vi "dlcTAF.vi"() -> ()   [LabVIEW 2019]
uses:
  <vilib>/DAQmx/write.llb/DAQmx Write (Digital 1D Bool NChan 1Samp 1Line).vi
  <vilib>/DAQmx/write.llb/DAQmx Write (Analog 1D DBL 1Chan NSamp).vi
  <vilib>/DAQmx/read.llb/DAQmx Read (Analog 2D I16 NChan NSamp).vi
  <vilib>/Analysis/baseanly.llb/Mean (DBL).vi
  Instance           1 17Saved   evtaf_amp .vi
  <vilib>/Utility/config.llb/Read Key (Path).vi
  <vilib>/Utility/config.llb/Read Key (String).vi
  <vilib>/Utility/config.llb/Read Key (I32).vi
  <vilib>/Utility/config.llb/Read Key (Double).vi
  <vilib>/Utility/config.llb/Read Key (U32).vi
  Instance           2 17Saved   evtaf_amp .vi
  Instance           3 17Saved   evtaf_amp .vi
  <vilib>/Utility/config.llb/Write Key (Path).vi
  <vilib>/Utility/config.llb/Write Key (String).vi
  <vilib>/Utility/config.llb/Write Key (Double).vi
  <vilib>/Utility/config.llb/Write Key (I32).vi
  <vilib>/Utility/config.llb/Write Key (U32).vi
  <vilib>/Utility/file.llb/Read Delimited Spreadsheet (DBL).vi
  <vilib>/DAQmx/create/channels.llb/DAQmx Create Channel (AO-Voltage-Basic).vi
  <vilib>/DAQmx/create/channels.llb/DAQmx Create Channel (DO-Digital Output).vi
  <vilib>/DAQmx/miscellaneous.llb/DAQmx Fill In Error Info.vi
  <vilib>/DAQmx/configure/timing.llb/DAQmx Timing (Sample Clock).vi
  <vilib>/DAQmx/configure/trigger.llb/DAQmx Start Trigger (Digital Edge).vi
  <vilib>/DAQmx/create/channels.llb/DAQmx Create Channel (AI-Voltage-Basic).vi
  <vilib>/Utility/config.llb/NI_LVConfig.lvlib
  <resource>/objmgr/daqmx.rc
  <vilib>/Analysis/NI_AALBase.lvlib
panel:
  in  "UDP_port":u16=53000
  in  "occurrence":refnum<k4>
  out "UDP_packet_contents":string="0"
  out "packet_timestamp_sec":dbl format="%#.10g"
  out "packet_latency_ms":dbl format="%#.10g"
  out "time_when_received_sec":dbl format="%#.10f"
  out "UDP Trig":bool
  out "UDP Packet Error":errorcluster
  out "RecSigs":bool[](array[boolean])
  in  "REC LED Pin":tag="Dev1/port0/line2"
  out "tic":dbl=16343.098892687482 format="%_19f"
  in  "REC Trig Pin":tag="Dev1/port0/line1"
  in  "Clock Source":tag="OnboardClock"
  in  "Slope Trig":bool
  out "Memory Lag":bool
  out "Prev Spike":i16[](array[numeric])
  in  "Threshold (mV)":sgl(slide)=4465.4087 min=-10000 max=10000 scale=-10000.0..10000.0
  out "DataBefTrig":i32=64000
  in  "Auto Trig Refrac?":bool=TRUE
  in  "Window (ms)":u16(slide)=101 min=1 max=2000 step=1 scale=1.0..2000.0
  in  "Trig Edge?":bool
  out "Max Voltage":dbl=10.0
  out "Syll Freqs":dbl[](array[numeric]) format="%#.5g"
  out "Targ Syll Freq (Hz)":dbl
  out "N Catch Esc":i16
  in  "Time Test?":bool
  out "Read dt":u32
  out "Trig Time":u32=282572892
  in  "AO Amp Fac":dbl=0.95 min=0.0 max=1.0 step=0.05
  in  "Amp Det Ch":i32
  out "N Detect":i32
  in  "Smth Fac":dbl=0.01
  out "Mean":dbl=-370.514489709558 format="%#.1f"
  in  "AmpClust":T1={"Min Freq(Hz)"=1000.0, "Max Freq(Hz)"=3500.0, "Amp TH"=100.0, "AmpMode"=1} {"AmpMode" items=["Below Hits", "Above Hits"]}
  in  "File State Ch":i32
  out "FreqVals":dbl[](array[numeric])=[0.0, 125.0, 250.0, 375.0, 500.0, 625.0, 750.0, 875.0, 1000.0, 1125.0, 1250.0, 1375.0, 1500.0, 1625.0, 1750.0, 1875.0, 2000.0, 2125.0, 2250.0, 2375.0, 2500.0, 2625.0, 2750.0, 2875.0, 3000.0, 3125.0, 3250.0, 3375.0, 3500.0, 3625.0, 3750.0, 3875.0, 4000.0, 4125.0, 4250.0, 4375.0, 4500.0, 4625.0, 4750.0, 4875.0, 5000.0, 5125.0, 5250.0, 5375.0, 5500.0, 5625.0, 5750.0, 5875.0, 6000.0, 6125.0, 6250.0, 6375.0, 6500.0, 6625.0, 6750.0, 6875.0, 7000.0, 7125.0, 7250.0, 7375.0, 7500.0, 7625.0, 7750.0, 7875.0, 8000.0, 8125.0, 8250.0, 8375.0, 8500.0, 8625.0, 8750.0, 8875.0, 9000.0, 9125.0, 9250.0, 9375.0, 9500.0, 9625.0, 9750.0, 9875.0, 10000.0, 10125.0, 10250.0, 10375.0, 10500.0, 10625.0, 10750.0, 10875.0, 11000.0, 11125.0, 11250.0, 11375.0, 11500.0, 11625.0, 11750.0, 11875.0, 12000.0, 12125.0, 12250.0, 12375.0, 12500.0, 12625.0, 12750.0, 12875.0, 13000.0, 13125.0, 13250.0, 13375.0, 13500.0, 13625.0, 13750.0, 13875.0, 14000.0, 14125.0, 14250.0, 14375.0, 14500.0, 14625.0, 14750.0, 14875.0, 15000.0, 15125.0, 15250.0, 15375.0, 15500.0, 15625.0, 15750.0, 15875.0]
  out "NFFT":i32=256
  in  "FreqClust":T2={"Min Freq(Hz)"=1000.0, "Max Freq(Hz)"=3500.0, "Freq TH Min(Hz)"=1000.0, "Freq TH Max(Hz)"=3500.0, "NBins"=3, "FreqMode"=2} {"FreqMode" items=["Below Hits", "Above Hits", "Between Hits", "Outside Hits"]}
  in  "Save Config":bool
  in  "Load Config":bool
  in  "Start":bool
  out "AO Len":dbl=0.5172126372 format="%#_4g"
  in  "WhichChan":i32=1
  out "Catch?":i32[](array[numeric])
  out "Catch Trial?":bool
  in  "Catch Trial\nFraction":dbl min=0.0 max=1.0 step=0.01 format="%#.2f"
  out "T Bef":dbl=2.0
  out "Reset Trig Error 2":errorcluster
  out "Reset Trig Error1":errorcluster
  out "Index":i32=60524
  out "DOtask":refnum<k21>
  in  "TAF Trig Out":tag="Dev1/port0/line7"
  out "AO task":refnum<k21>
  out "AO Nwrtn":u32=22579
  out "Catch Song?":bool
  in  "Catch Song\nFraction":dbl min=0.0 max=1.0 step=0.01 format="%#.2f"
  out "Neural Data":sgl[](graph)=[-115.35997, -115.05479, -115.05479, -115.05479]
  out "Song Data":i16[](graph)=[-310, -338, -330, -332]
  in  "Plot2":bool=TRUE
  in  "Sound Rates":dbl[](array[numeric])=[11025.0, 22050.0, 44100.0] format="%.2f"
  out "AI Actual Update":dbl=3.125e-05 format="%.2f"
  out "Outfile RefNum":refnum<file>
  out "Sound Format":T3={"Sound Quality"=0, "Rate"=2, "Resolution"=1} {"Resolution" items=["8 bit", "16 bit"]; "Rate" items=["11025", "22050", "44100", "8000"]; "Sound Quality" items=["Mono", "Setero"]}
  out "Templates":sgl[][](array[numeric])=[[0.0, 0.0], [0.0, 0.0], [0.0, 0.0], [0.0, 0.0], [0.0, 0.0], [0.0, 0.0], [0.0556644, 0.0254043], [0.020632, 0.00778995], [0.0529074, 0.0129611], [0.0872023, 0.034105], [0.0454044, 0.0175483], [0.0283851, 0.00925169], [0.0256533, 0.00647604], [0.0305833, 0.0073634], [0.0303148, 0.0114906], [0.035281, 0.0113772], [0.0342556, 0.0117177], [0.0312334, 0.0107575], [0.0684019, 0.0328105], [0.0974883, 0.35804], [0.304953, 1.0], [1.0, 0.259667], [0.150841, 0.0228862], [0.0366788, 0.0096238], [0.0231339, 0.00747089], [0.0197387, 0.00936122], [0.0130916, 0.00779655], [0.0160134, 0.013076], [0.0128113, 0.0141189], [0.0156363, 0.00924646], [0.0137237, 0.00802244], [0.0162737, 0.00636405], [0.0302698, 0.0102784], [0.0262628, 0.00772131], [0.0216469, 0.00680912], [0.0281085, 0.00714835], [0.0334301, 0.0134141], [0.0582892, 0.0229925], [0.0730454, 0.0783954], [0.139458, 0.225434], [0.175723, 0.211888], [0.571615, 0.100956], [0.986431, 0.0383641], [0.669511, 0.0190024], [0.366205, 0.0170195], [0.15179, 0.0120307], [0.0850952, 0.0156807], [0.0531273, 0.0166329], [0.0353153, 0.0153677], [0.0207535, 0.0130318], [0.0176546, 0.0120725], [0.0180874, 0.0164731], [0.0180358, 0.0174649], [0.0199549, 0.019393], [0.0156083, 0.0173286], [0.0149243, 0.0267737], [0.0148128, 0.0672004], [0.0177527, 0.207942], [0.0190198, 0.501856], [0.0232154, 0.889056], [0.0264518, 0.892834], [0.0372134, 0.606768], [0.0570822, 0.201655], [0.0799642, 0.0537564], [0.0517915, 0.0324652], [0.030705, 0.0160809], [0.0173904, 0.0131532], [0.00948186, 0.0108228], [0.00763086, 0.00893009], [0.00472818, 0.0073349], [0.00463126, 0.00813084], [0.004089, 0.00965328], [0.00311063, 0.00770917], [0.00342832, 0.00813488], [0.00365656, 0.0122865], [0.00381178, 0.0217128], [0.00333337, 0.0392938], [0.00357412, 0.0813244], [0.00363441, 0.150175], [0.00453097, 0.175109], [0.00185524, 0.0634255], [0.000370271, 0.00192084], [0.000370235, 0.000379918], [0.000370235, 0.000216318], [0.000370235, 0.000191697], [0.000370235, 0.000189425], [0.000370235, 0.000189382], [0.000370235, 0.000189382], [0.000370235, 0.000189382], [0.000370235, 0.000189382], [0.000370235, 0.000189382], [0.000370235, 0.000189382], [0.000370235, 0.000189382], [0.000370235, 0.000189382], [0.000370235, 0.000189382], [0.000370235, 0.000189382], [0.000370235, 0.000189382], [0.000370235, 0.000189382], [0.000370235, 0.000189382], [0.000370235, 0.000189382], [0.000370235, 0.000189382], [0.000370235, 0.000189382], [0.000370235, 0.000189382], [0.000370235, 0.000189382], [0.000370235, 0.000189382], [0.000370235, 0.000189382], [0.000370235, 0.000189382], [0.000370235, 0.000189382], [0.000370235, 0.000189382], [0.000370235, 0.000189382], [0.000370235, 0.000189382], [0.000370235, 0.000189382], [0.000370235, 0.000189382], [0.000370235, 0.000189382], [0.000370235, 0.000189382], [0.000370235, 0.000189382], [0.000370235, 0.000189382], [0.000370235, 0.000189382], [0.000370235, 0.000189382], [0.000370235, 0.000189382], [0.000370235, 0.000189382], [0.000370235, 0.000189382], [0.000370235, 0.000189382], [0.000370235, 0.000189382], [0.000370235, 0.000189382], [0.000370235, 0.000189382], [0.000370235, 0.000189382], [0.000370235, 0.000189382]] format="%.2f"
  in  "FFT Thresholds":dbl[](array[numeric])=[2.2, 2.5] format="%.2f"
  out "Trig Times":dbl[](array[numeric]) format="%.2f"
  in  "Temp Out":dbl[](array[numeric]) format="%.2f"
  in  "Counter Rng":T4(array[cluster])=[{"Min"=2, "Max"=16, "Not"=FALSE, "Mode"=FALSE, "BTAFmin"=0, "AND/OR"=FALSE}, {"Min"=2, "Max"=8, "Not"=FALSE, "Mode"=TRUE, "BTAFmin"=0, "AND/OR"=FALSE}]
  in  "Plot":bool=TRUE
  out "Sound":dbl[](array[numeric]) format="%.2e"
  in  "File Open?":bool
  out "Counters":u32[](array[numeric])=[5429, 0]
  out "Current File":path=path "C:/ExperimentalBirds/EvTAF_Troubleshooting/bl26br1_exe/bl26br1_240519_1958.00.cbin"
  in  "Output Sound":path=path "C:/EvTAF2018.exe/playbacks/whitenoise_512_ms.wav"
  in  "Templates":path=path "C:/ExperimentalBirds/EvTAF_Troubleshooting/bl26br1_x_template"
  in  "Output Path":path=path "C:/ExperimentalBirds/EvTAF_Troubleshooting/bl26br1_exe"
  in  "Bird Name":string="bl26br1"
  out "First Dat":bool=TRUE
  out "Trigger":bool
  out "N Trig":u32
  in  "Manual Trigger":bool
  out "Silence T":dbl=3.0 format="%.1f"
  out "Buffer Size":i32=128000
  out "T snc trig":dbl=277.8913749995362 format="%.1f"
  out "N AI Chan":i32=2
  out "Total Data T":dbl format="%.1f"
  in  "Trig Refrac(s)":dbl=0.5172126372 format="%.3f"
  in  "Min Data Time":dbl=5.0 format="%.2f"
  out "N Files":i16=21
  in  "Data Aft Trig(s)":dbl=2.0 format="%.2f"
  in  "Data Bef Trig(s)":dbl=2.0 format="%.2f"
  in  "stop":bool
  in  "Raw Threshold":i32(slide)=500 min=0 step=1 scale=0.0..40000.0
  out "AO Started?":bool=TRUE
  out "N Read":i32=4
  in  "Syll Det Ch":i32
  out "AI Rate":dbl=32000.0 format="%#.12f"
  out "Real AO Rate":sgl=44091.71 format="%#.2f"
  in  "Analog Input Config":T5={"AI Channels"="Dev1/ai0:1", "Scan Rate(kHz)"=32.0, "Min Voltage"=-10, "Max Voltage"=10, "Chan Name"="AI"} {"Max Voltage" items=["10"=10, "5"=5, "1"=1]; "Min Voltage" items=["-10"=-10, "-5"=-5, "-1"=-1]; "Scan Rate(kHz)" format="%.2f"}
  in  "Analog Output Config":T6={"Min Voltage"=-10, "Max Voltage"=10, "AO Channels"="Dev1/ao0", "Chan Name"="AO", "TAF Trig In"="/Dev1/PFI1"} {"Max Voltage" items=["10"=10, "5"=5, "1"=1]; "Min Voltage" items=["-10"=-10, "-5"=-5, "-1"=-1]}
  out "Too Much Data":bool
  out "Threshold Error":errorcluster
  out "AI Error":errorcluster
  out "AO Error":errorcluster
  # "Digital IO Config"
  # "Raw Song"
  # "Neural Data"
  # "-"
  # "+"
  # "F"
  # "T"
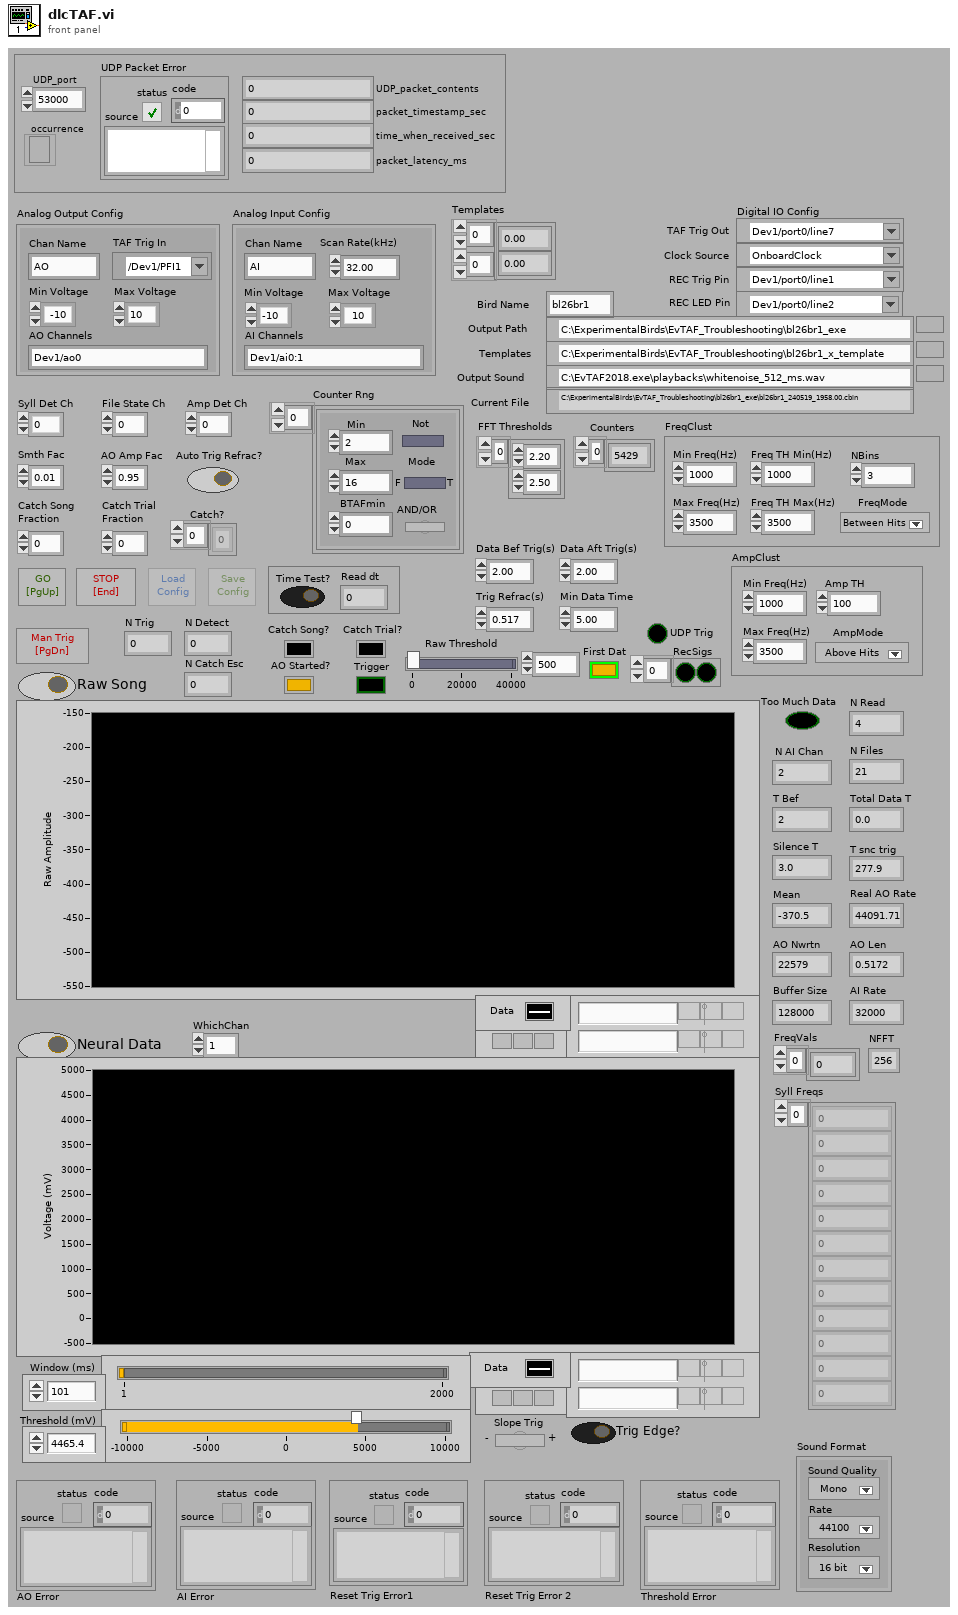
[diagram p1: front panel]
types:
  T1 = cluster{"Min Freq(Hz)":dbl, "Max Freq(Hz)":dbl, "Amp TH":dbl, "AmpMode":u16}
  T2 = cluster{"Min Freq(Hz)":dbl, "Max Freq(Hz)":dbl, "Freq TH Min(Hz)":dbl, "Freq TH Max(Hz)":dbl, "NBins":i32, "FreqMode":u16}
  T3 = cluster{"Sound Quality":u16, "Rate":u16, "Resolution":u16}
  T4 = cluster{"Min":i16, "Max":i16, "Not":bool, "Mode":bool, "BTAFmin":i16, "AND/OR":bool}[]
  T5 = cluster{"AI Channels":string, "Scan Rate(kHz)":dbl, "Min Voltage":i8, "Max Voltage":i8, "Chan Name":string}
  T6 = cluster{"Min Voltage":i8, "Max Voltage":u16, "AO Channels":string, "Chan Name":string, "TAF Trig In":tag}
  T7 = cluster{"Min":i16, "Max":i16, "Not":bool, "Mode":bool, i32, bool}[]
  T8 = typedef "NI_LVConfig.lvlib/Config Data RefNum.ctl" = refnum<k1>
  T9 = typedef "Sound Format.ctl" = cluster{"sound quality":enum16{"mono", "stereo"}, "rate":enum16{"11025", "22050", "44100", "8000"}, "bits per sample":enum16{"8 bit", "16 bit"}}
  T10 = cluster{"Data Bef Trig(s)":dbl, "Data Aft Trig(s)":dbl, "FFT Thresholds":dbl[], "Output Sound":path}
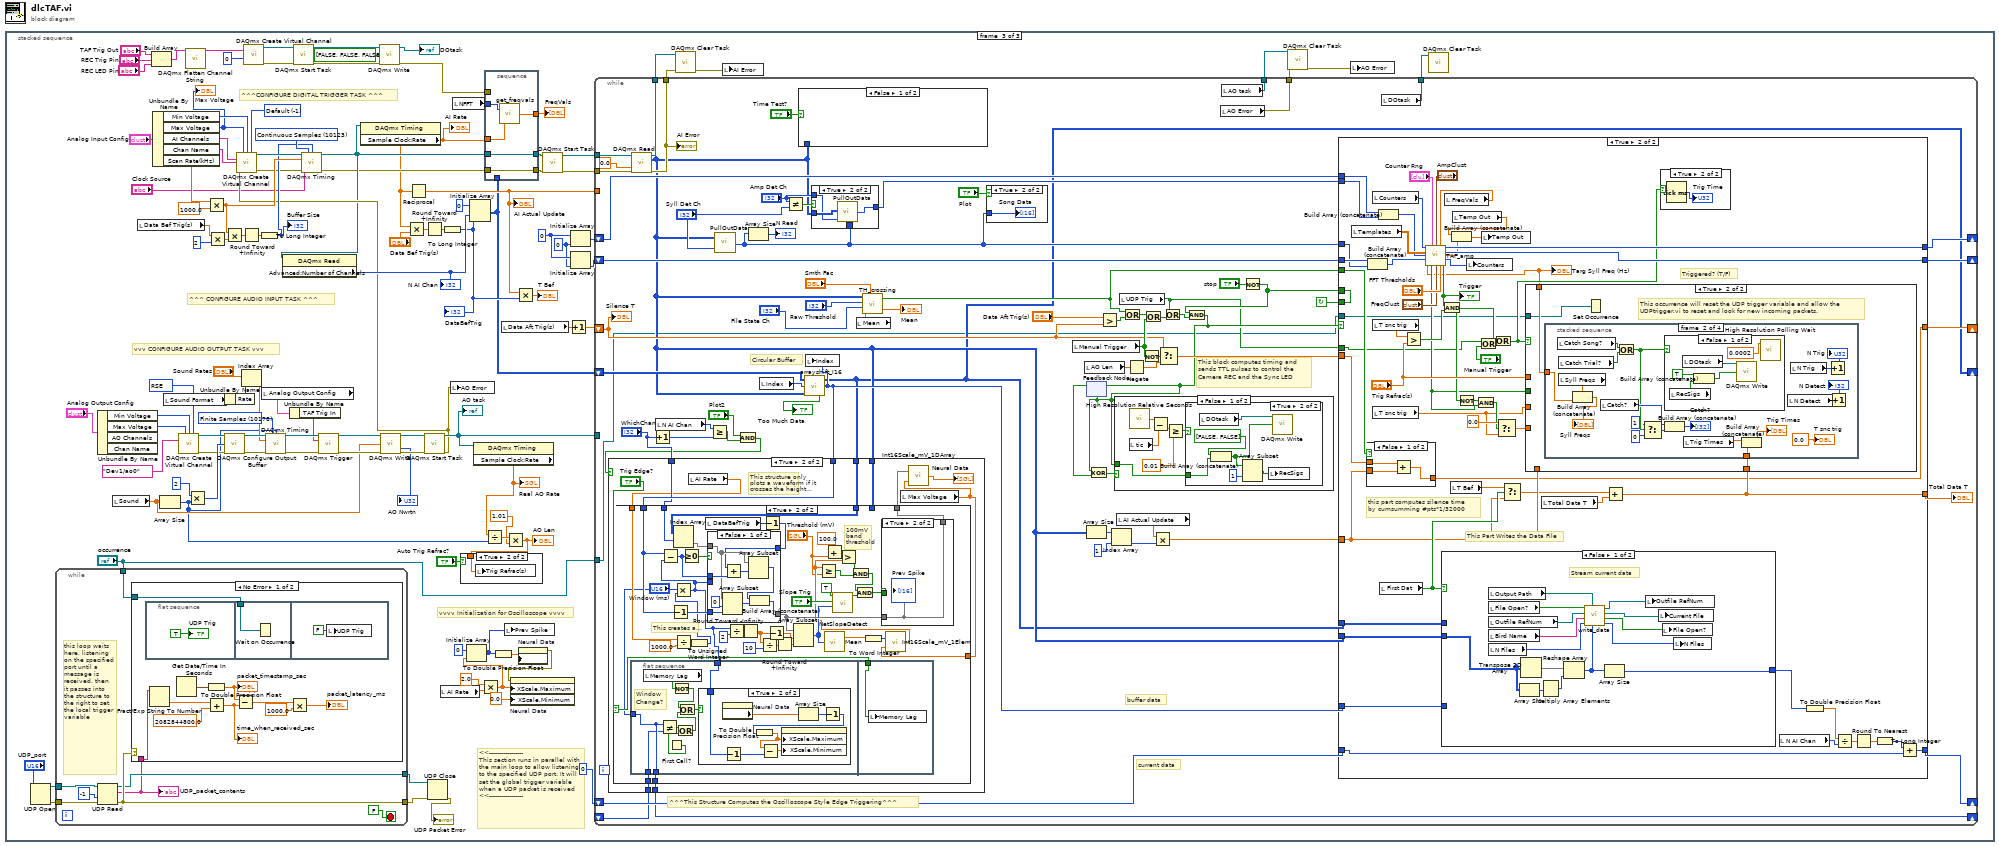
[diagram p0: block diagram]
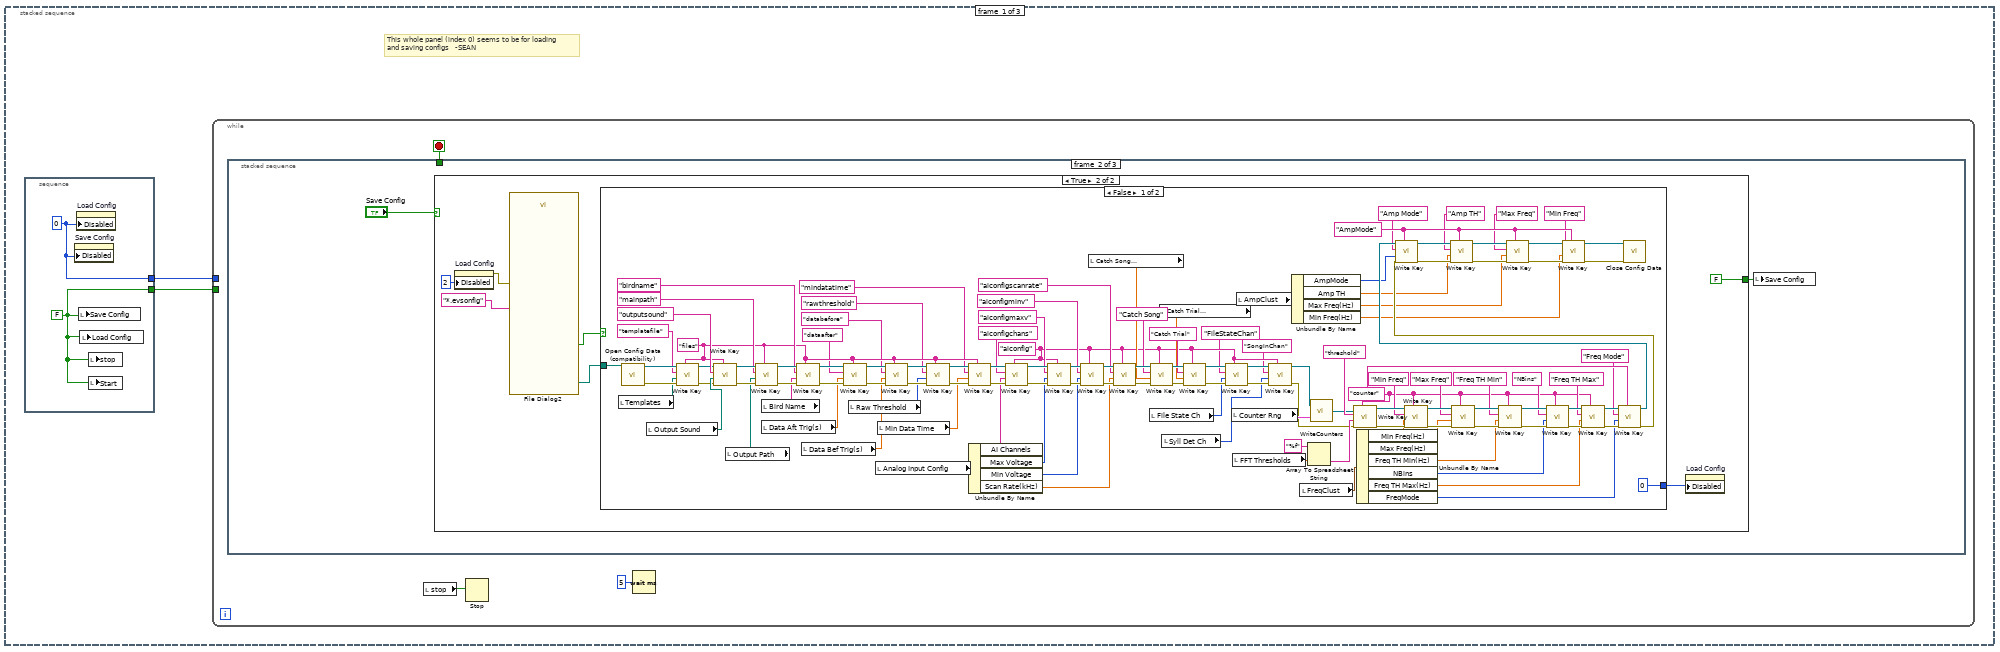
[diagram p2: hidden frame]
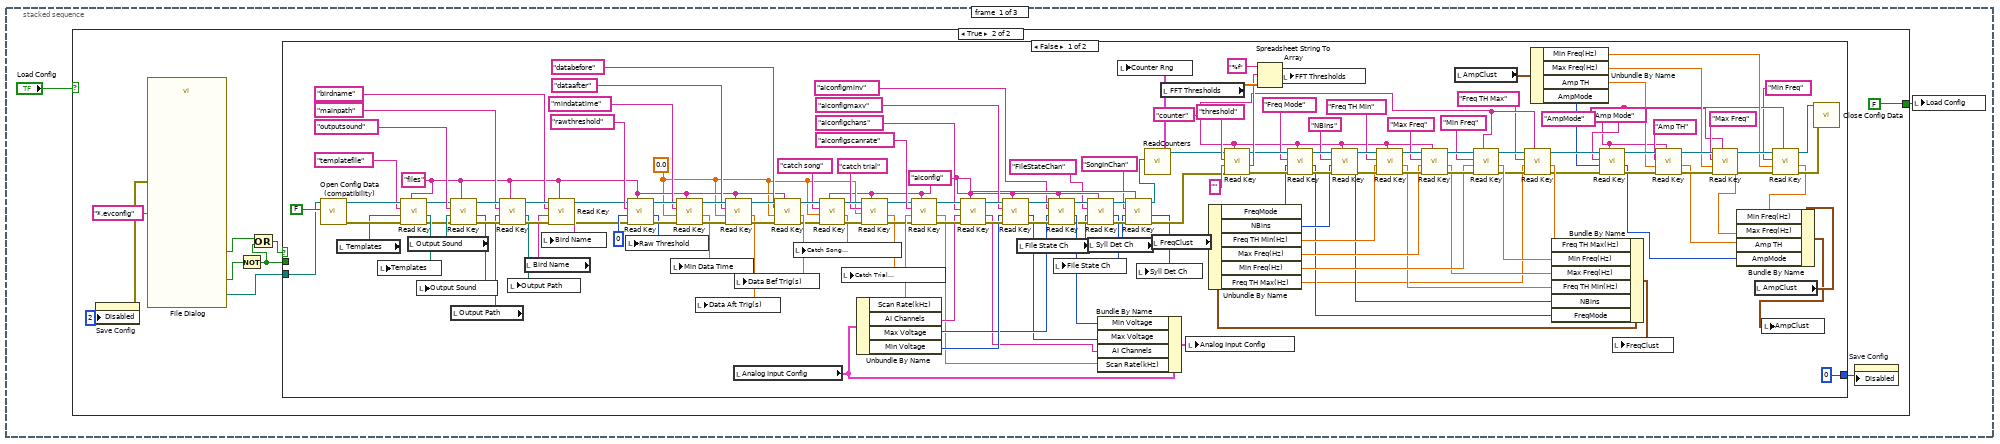
[diagram p3: hidden frame]
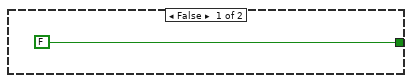
[diagram p4: hidden frame]
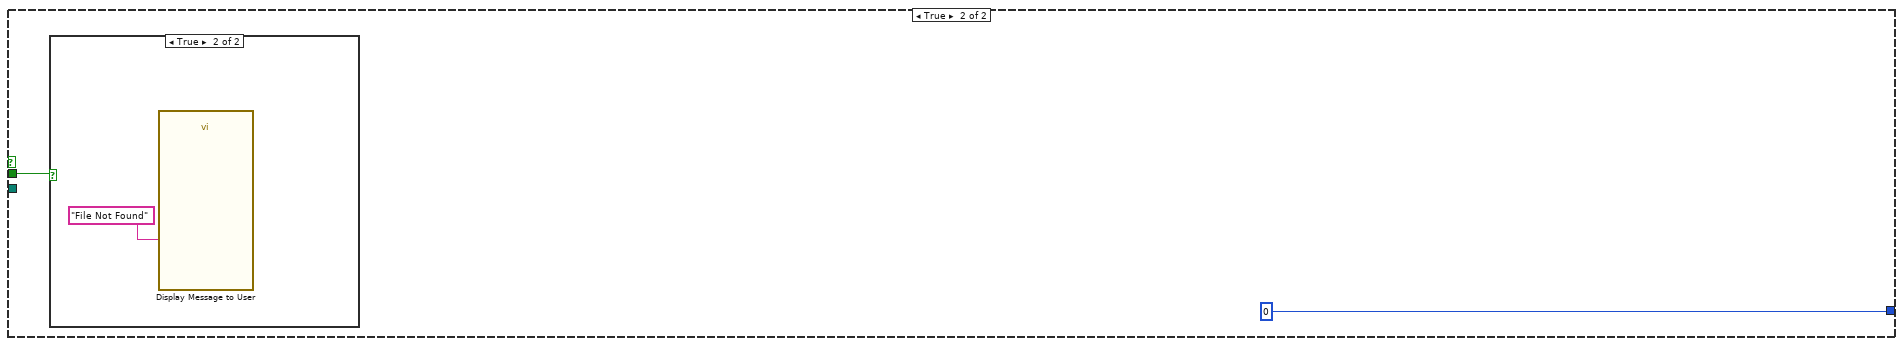
[diagram p5: hidden frame]
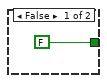
[diagram p7: hidden frame]
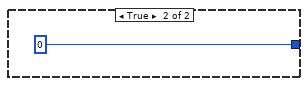
[diagram p8: hidden frame]
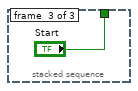
[diagram p9: hidden frame]
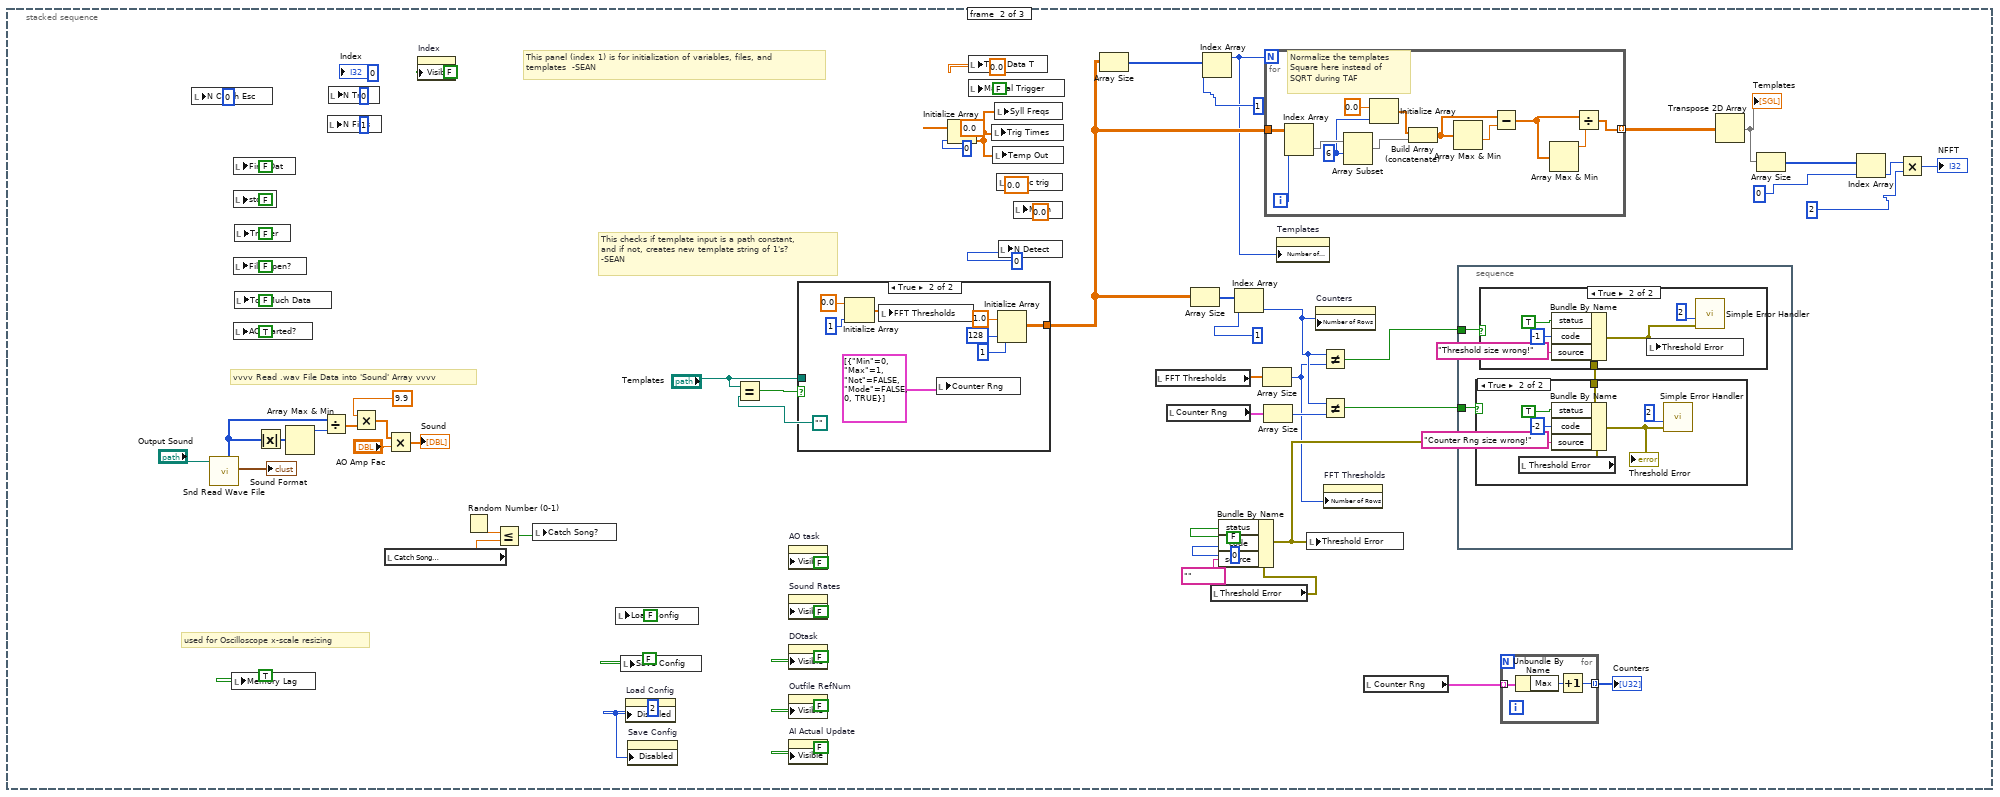
[diagram p10: hidden frame]
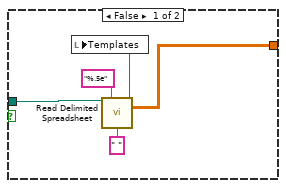
[diagram p11: hidden frame]
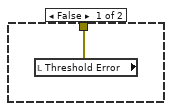
[diagram p12: hidden frame]
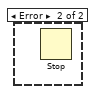
[diagram p14: hidden frame]
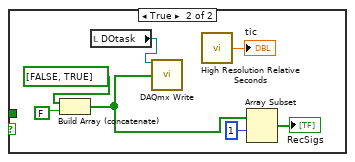
[diagram p17: hidden frame]
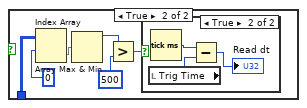
[diagram p18: hidden frame]
diagram:
  n1 = stacked-sequence {
    frame #0 {
      # "This whole panel (index 0) seems to be for loading\nand saving configs   -SEAN"
      n2 = stacked-sequence {
        tunnel: [w4] -> w2
        tunnel: [w3] -> w1
        frame #0 {
          w3 = FALSE ("Save Config")
          w4 = u8 0 ("Disabled")
          n3 = property on="Save Config" class="Bool (strict)"("Disabled"=w4) -> ()  [unwired: 2 in, 2 out]
          n4 = property on="Load Config" class="Bool (strict)"("Disabled"=w4) -> ()  [unwired: 2 in, 2 out]
          n5 = local write "Save Config"(w3) -> ()
          n6 = local write "Load Config"(w3) -> ()
          n7 = local write "stop"(w3) -> ()
          n8 = local write "Start"(w3) -> ()
        }
      }
      n9 = while {
        tunnel: w2 -> [_]
        tunnel: w1 -> [_]
        stop <- w7 stop-if-true
        n10 = stacked-sequence {
          tunnel: [_ _ "Start"] -> w7
          frame #0 {
            n11 = case shown="True" "Load Config" {
              tunnel: [FALSE ("Load Config") FALSE ("Load Config")] -> w8
              frame False {
              }
              frame True {
                n12 = property on="Save Config" class="Bool (strict)"("Disabled"=u8 2) -> (error out=w13:errorcluster)  [unwired: 2 in, 1 out]
                n13 = call "File Dialog"("prompt"="*.evconfig" ("pattern label"), "error in"=w13) -> ("selected path"=w15:path, "exists"=w19:bool, "cancelled"=w18:bool)  [unwired: 10 in, 1 out]
                n14 = Not(x=w19) -> (.not. x?=w16:bool)
                n15 = Or(x=w18, y=w16) -> (x .or. y?=w17:bool)
                n16 = case shown="False" w17 {
                  tunnel: w16 -> [_ w174]
                  tunnel: w15 -> [w118 _]
                  tunnel: [0 0] -> w12
                  frame False {
                    w22 = "AmpMode" ("key")
                    w75 = "counter"
                    w38 = "aiconfig" ("section")
                    w113 = "files" ("section")
                    w63 = 0.0
                    n17 = call <vilib>:"Open Config Data (compatibility).vi"("create file if necessary (T)"=FALSE ("create file if necessary? (T)"), "configuration file path"=w118) -> ("error out"=w170:errorcluster, "refnum"=w171:T8)  [unwired: 7 in, 1 out]
                    n18 = local read "Templates"() -> (w145:path)
                    n19 = call-poly <vilib>:"Read Key.vi"("section"=w113, "error in (no error)"=w170, "default value"=w145, "key"="templatefile", "refnum"=w171) -> ("error out"=w116:errorcluster, "value"=w146:path, "refnum out"=w117:T8)  [unwired: 3 in, 1 out]
                    n20 = local write "Templates"(w146) -> ()
                    n21 = local read "Output Sound"() -> (w149:path)
                    n22 = call-poly <vilib>:"Read Key.vi"("section"=w113, "error in (no error)"=w116, "default value"=w149, "key"="outputsound", "refnum"=w117) -> ("error out"=w163:errorcluster, "value"=w148:path, "refnum out"=w169:T8)  [unwired: 3 in, 1 out]
                    n23 = local write "Output Sound"(w148) -> ()
                    n24 = local read "Output Path"() -> (w151:path)
                    n25 = call-poly <vilib>:"Read Key.vi"("section"=w113, "error in (no error)"=w163, "default value"=w151, "key"="mainpath", "refnum"=w169) -> ("error out"=w162:errorcluster, "value"=w150:path, "refnum out"=w168:T8)  [unwired: 3 in, 1 out]
                    n26 = local write "Output Path"(w150) -> ()
                    n27 = local read "Bird Name"() -> (w153:string)
                    n28 = call-poly <vilib>:"Read Key.vi"("section"=w113, "error in (no error)"=w162, "default value"=w153, "key"="birdname", "refnum"=w168) -> ("error out"=w112:errorcluster, "value"=w152:string, "refnum out"=w114:T8)  [unwired: 3 in, 1 out]
                    n29 = local write "Bird Name"(w152) -> ()
                    n30 = call-poly <vilib>:"Read Key.vi"("section"=w113, "error in (no error)"=w112, "default value"=0, "key"="rawthreshold", "refnum"=w114) -> ("error out"=w160:errorcluster, "value"=w136:i32, "refnum out"=w166:T8)  [unwired: 3 in, 1 out]
                    n31 = local write "Raw Threshold"(w136) -> ()
                    n32 = call-poly <vilib>:"Read Key.vi"("section"=w113, "error in (no error)"=w160, "default value"=w63, "key"="mindatatime", "refnum"=w166) -> ("error out"=w159:errorcluster, "value"=w138:dbl, "refnum out"=w165:T8)  [unwired: 3 in, 1 out]
                    n33 = local write "Min Data Time"(w138) -> ()
                    n34 = call-poly <vilib>:"Read Key.vi"("section"=w113, "error in (no error)"=w159, "default value"=w63, "key"="dataafter", "refnum"=w165) -> ("error out"=w158:errorcluster, "value"=w139:dbl, "refnum out"=w164:T8)  [unwired: 3 in, 1 out]
                    n35 = local write "Data Aft Trig(s)"(w139) -> ()
                    n36 = local read "Analog Input Config"() -> (w123:T5)
                    n37 = call-poly <vilib>:"Read Key.vi"("section"=w113, "error in (no error)"=w158, "default value"=w63, "key"="databefore", "refnum"=w164) -> ("error out"=w70:errorcluster, "value"=w140:dbl, "refnum out"=w71:T8)  [unwired: 3 in, 1 out]
                    n38 = local write "Data Bef Trig(s)"(w140) -> ()
                    n39 = call-poly <vilib>:"Read Key.vi"("section"=w38, "error in (no error)"=w70, "default value"=w63, "key"="catch song", "refnum"=w71) -> ("error out"=w66:errorcluster, "value"=w62:dbl, "refnum out"=w68:T8)  [unwired: 3 in, 1 out]
                    n40 = local write "Catch Song\nFraction"(w62) -> ()
                    n41 = Unbundle By Name(w123) -> ("Scan Rate(kHz)"=w128:dbl, "AI Channels"=w127:string, "Max Voltage"=w126:i8, "Min Voltage"=w125:i8)
                    n42 = call-poly <vilib>:"Read Key.vi"("section"=w38, "error in (no error)"=w66, "default value"=w63, "key"="catch trial", "refnum"=w68) -> ("error out"=w65:errorcluster, "value"=w61:dbl, "refnum out"=w67:T8)  [unwired: 3 in, 1 out]
                    n43 = local write "Catch Trial\nFraction"(w61) -> ()
                    n44 = call-poly <vilib>:"Read Key.vi"("section"=w38, "error in (no error)"=w65, "default value"=w128, "key"="aiconfigscanrate", "refnum"=w67) -> ("error out"=w161:errorcluster, "value"=w119:dbl, "refnum out"=w167:T8)  [unwired: 3 in, 1 out]
                    n45 = call-poly <vilib>:"Read Key.vi"("section"=w38, "error in (no error)"=w161, "default value"=w127, "key"="aiconfigchans", "refnum"=w167) -> ("error out"=w132:errorcluster, "value"=w120:string, "refnum out"=w135:T8)  [unwired: 3 in, 1 out]
                    n46 = call-poly <vilib>:"Read Key.vi"("section"=w38, "error in (no error)"=w132, "default value"=w126, "key"="aiconfigmaxv", "refnum"=w135) -> ("error out"=w133:errorcluster, "value"=w121:i32, "refnum out"=w134:T8)  [unwired: 3 in, 1 out]
                    n47 = local read "File State Ch"() -> (w29:i32)
                    n48 = call-poly <vilib>:"Read Key.vi"("section"=w38, "error in (no error)"=w133, "default value"=w125, "key"="aiconfigminv", "refnum"=w134) -> ("error out"=w33:errorcluster, "value"=w122:i32, "refnum out"=w39:T8)  [unwired: 3 in, 1 out]
                    n49 = local read "Syll Det Ch"() -> (w27:i32)
                    n50 = call-poly <vilib>:"Read Key.vi"("section"=w38, "error in (no error)"=w33, "default value"=w29, "key"="FileStateChan", "refnum"=w39) -> ("error out"=w34:errorcluster, "value"=w28:i32, "refnum out"=w37:T8)  [unwired: 3 in, 1 out]
                    n51 = local write "File State Ch"(w28) -> ()
                    n52 = Bundle By Name(cluster=w123, "Min Voltage"=w122, "Max Voltage"=w121, "AI Channels"=w120, "Scan Rate(kHz)"=w119) -> (w124:T5)
                    n53 = call-poly <vilib>:"Read Key.vi"("section"=w38, "error in (no error)"=w34, "default value"=w27, "key"="SongInChan", "refnum"=w37) -> ("error out"=w35:errorcluster, "value"=w26:i32, "refnum out"=w36:T8)  [unwired: 3 in, 1 out]
                    n54 = local write "Syll Det Ch"(w26) -> ()
                    n55 = call "ReadCounters.vi"("refnum"=w36) -> ("refnum out"=w80:T8, "Counters"=w79:T4)
                    n56 = local write "Counter Rng"(w79) -> ()
                    n57 = local read "FreqClust"() -> (w96:T2)
                    n58 = local read "FFT Thresholds"() -> (w147:dbl[])
                    n59 = local write "Analog Input Config"(w124) -> ()
                    n60 = Unbundle By Name(w96) -> ("FreqMode"=w85:u16, "NBins"=w86:i32, "Freq TH Min(Hz)"=w87:dbl, "Max Freq(Hz)"=w88:dbl, "Min Freq(Hz)"=w94:dbl, "Freq TH Max(Hz)"=w73:dbl)
                    n61 = call-poly <vilib>:"Read Key.vi"("section"=w75, "error in (no error)"=w35, "default value"="", "key"="threshold", "refnum"=w80) -> ("error out"=w107:errorcluster, "value"=w109:string, "refnum out"=w102:T8)  [unwired: 3 in, 1 out]
                    n62 = Spreadsheet String To Array(format string="%f", spreadsheet string=w109, array type (2D Dbl)=w147) -> (array=w78:dbl[])  [unwired: 1 in]
                    n63 = local write "FFT Thresholds"(w78) -> ()
                    n64 = call-poly <vilib>:"Read Key.vi"("section"=w75, "error in (no error)"=w107, "default value"=w85, "key"="Freq Mode", "refnum"=w102) -> ("error out"=w106:errorcluster, "value"=w84:u32, "refnum out"=w101:T8)  [unwired: 3 in, 1 out]
                    n65 = call-poly <vilib>:"Read Key.vi"("section"=w75, "error in (no error)"=w106, "default value"=w86, "key"="NBins", "refnum"=w101) -> ("error out"=w105:errorcluster, "value"=w83:i32, "refnum out"=w100:T8)  [unwired: 3 in, 1 out]
                    n66 = call-poly <vilib>:"Read Key.vi"("section"=w75, "error in (no error)"=w105, "default value"=w87, "key"="Freq TH Min", "refnum"=w100) -> ("error out"=w104:errorcluster, "value"=w82:dbl, "refnum out"=w99:T8)  [unwired: 3 in, 1 out]
                    n67 = call-poly <vilib>:"Read Key.vi"("section"=w75, "error in (no error)"=w104, "default value"=w88, "key"="Max Freq", "refnum"=w99) -> ("error out"=w103:errorcluster, "value"=w81:dbl, "refnum out"=w98:T8)  [unwired: 3 in, 1 out]
                    n68 = local read "AmpClust"() -> (w60:T1)
                    n69 = call-poly <vilib>:"Read Key.vi"("section"=w75, "error in (no error)"=w103, "default value"=w94, "key"="Min Freq", "refnum"=w98) -> ("error out"=w76:errorcluster, "value"=w95:dbl, "refnum out"=w77:T8)  [unwired: 3 in, 1 out]
                    n70 = call-poly <vilib>:"Read Key.vi"("section"=w75, "error in (no error)"=w76, "default value"=w73, "key"="Freq TH Max", "refnum"=w77) -> ("error out"=w54:errorcluster, "value"=w72:dbl, "refnum out"=w59:T8)  [unwired: 3 in, 1 out]
                    n71 = Unbundle By Name(w60) -> ("Min Freq(Hz)"=w46:dbl, "Max Freq(Hz)"=w47:dbl, "Amp TH"=w48:dbl, "AmpMode"=w49:u16)
                    n72 = Bundle By Name(cluster=w96, "Freq TH Max(Hz)"=w72, "Min Freq(Hz)"=w95, "Max Freq(Hz)"=w81, "Freq TH Min(Hz)"=w82, "NBins"=w83, "FreqMode"=w84) -> (w97:T2)
                    n73 = call-poly <vilib>:"Read Key.vi"("section"=w22, "error in (no error)"=w54, "default value"=w49, "key"="Amp Mode" ("section"), "refnum"=w59) -> ("error out"=w53:errorcluster, "value"=w43:u32, "refnum out"=w58:T8)  [unwired: 3 in, 1 out]
                    n74 = local write "FreqClust"(w97) -> ()
                    n75 = call-poly <vilib>:"Read Key.vi"("section"=w22, "error in (no error)"=w53, "default value"=w48, "key"="Amp TH" ("section"), "refnum"=w58) -> ("error out"=w52:errorcluster, "value"=w42:dbl, "refnum out"=w57:T8)  [unwired: 3 in, 1 out]
                    n76 = call-poly <vilib>:"Read Key.vi"("section"=w22, "error in (no error)"=w52, "default value"=w47, "key"="Max Freq" ("section"), "refnum"=w57) -> ("error out"=w51:errorcluster, "value"=w41:dbl, "refnum out"=w56:T8)  [unwired: 3 in, 1 out]
                    n77 = local read "AmpClust"() -> (w45:T1)
                    n78 = call-poly <vilib>:"Read Key.vi"("section"=w22, "error in (no error)"=w51, "default value"=w46, "key"="Min Freq" ("section"), "refnum"=w56) -> ("error out"=w50:errorcluster, "value"=w40:dbl, "refnum out"=w55:T8)  [unwired: 3 in, 1 out]
                    n79 = Bundle By Name(cluster=w45, "Min Freq(Hz)"=w40, "Max Freq(Hz)"=w41, "Amp TH"=w42, "AmpMode"=w43) -> (w44:T1)
                    n80 = local write "AmpClust"(w44) -> ()
                    n81 = call <vilib>:"Close Config Data.vi"("error in (no error)"=w50, "refnum"=w55) -> ()  [unwired: 8 in, 2 out]
                  }
                  frame True {
                    n82 = case shown="True" w174 {
                      frame False {
                      }
                      frame True {
                        n83 = call "Display Message to User"("Message"="File Not Found") -> ()  [unwired: 9 in, 2 out]
                      }
                    }
                  }
                }
                n84 = property on="Save Config" class="Bool (strict)"("Disabled"=w12) -> ()  [unwired: 2 in, 2 out]
              }
            }
            n85 = local write "Load Config"(w8) -> ()
          }
          frame #1 {
            n86 = case shown="True" "Save Config" {
              tunnel: [FALSE FALSE] -> w176
              frame False {
              }
              frame True {
                n87 = property on="Load Config" class="Bool (strict)"("Disabled"=u8 2) -> (error out=w182:errorcluster)  [unwired: 2 in, 1 out]
                n88 = call "File Dialog2"("error in"=w182, "pattern label"="*.evsonfig") -> ("selected path"=w183:path, "cancelled"=w184:bool)  [unwired: 10 in, 2 out]
                n89 = case shown="False" w184 {
                  tunnel: w183 -> [w308 _]
                  tunnel: [u8 0 u8 0] -> w180
                  frame False {
                    w190 = "AmpMode" ("key")
                    w228 = "counter"
                    w195 = "aiconfig" ("section")
                    w277 = "files" ("section")
                    n90 = local read "Templates"() -> (w288:path)
                    n91 = call <vilib>:"Open Config Data (compatibility).vi"("configuration file path"=w308) -> ("error out"=w300:errorcluster, "refnum"=w307:T8)  [unwired: 8 in, 1 out]
                    n92 = local read "Output Sound"() -> (w286:path)
                    n93 = call-poly <vilib>:"Write Key.vi"("section"=w277, "error in (no error)"=w300, "value"=w288, "key"="templatefile", "refnum"=w307) -> ("error out"=w252:errorcluster, "refnum out"=w253:T8)  [unwired: 4 in, 1 out]
                    n94 = call-poly <vilib>:"Write Key.vi"("section"=w277, "error in (no error)"=w252, "value"=w286, "key"="outputsound", "refnum"=w253) -> ("error out"=w299:errorcluster, "refnum out"=w306:T8)  [unwired: 4 in, 1 out]
                    n95 = local read "Output Path"() -> (w285:path)
                    n96 = call-poly <vilib>:"Write Key.vi"("section"=w277, "error in (no error)"=w299, "value"=w285, "key"="mainpath", "refnum"=w306) -> ("error out"=w298:errorcluster, "refnum out"=w305:T8)  [unwired: 4 in, 1 out]
                    n97 = local read "Bird Name"() -> (w284:string)
                    n98 = local read "Data Aft Trig(s)"() -> (w272:dbl)
                    n99 = call-poly <vilib>:"Write Key.vi"("section"=w277, "error in (no error)"=w298, "value"=w284, "key"="birdname", "refnum"=w305) -> ("error out"=w278:errorcluster, "refnum out"=w279:T8)  [unwired: 4 in, 1 out]
                    n100 = local read "Data Bef Trig(s)"() -> (w271:dbl)
                    n101 = call-poly <vilib>:"Write Key.vi"("section"=w277, "error in (no error)"=w278, "value"=w272, "key"="dataafter", "refnum"=w279) -> ("error out"=w297:errorcluster, "refnum out"=w304:T8)  [unwired: 4 in, 1 out]
                    n102 = local read "Raw Threshold"() -> (w270:i32)
                    n103 = local read "Analog Input Config"() -> (w260:T5)
                    n104 = local read "Min Data Time"() -> (w269:dbl)
                    n105 = call-poly <vilib>:"Write Key.vi"("section"=w277, "error in (no error)"=w297, "value"=w271, "key"="databefore", "refnum"=w304) -> ("error out"=w296:errorcluster, "refnum out"=w303:T8)  [unwired: 4 in, 1 out]
                    n106 = call-poly <vilib>:"Write Key.vi"("section"=w277, "error in (no error)"=w296, "value"=w270, "key"="rawthreshold", "refnum"=w303) -> ("error out"=w295:errorcluster, "refnum out"=w302:T8)  [unwired: 4 in, 1 out]
                    n107 = call-poly <vilib>:"Write Key.vi"("section"=w277, "error in (no error)"=w295, "value"=w269, "key"="mindatatime", "refnum"=w302) -> ("error out"=w294:errorcluster, "refnum out"=w301:T8)  [unwired: 4 in, 1 out]
                    n108 = Unbundle By Name(w260) -> ("AI Channels"=w259:string, "Max Voltage"=w258:i8, "Min Voltage"=w257:i8, "Scan Rate(kHz)"=w256:dbl)
                    n109 = call-poly <vilib>:"Write Key.vi"("section"=w195, "error in (no error)"=w294, "value"=w259, "key"="aiconfigchans", "refnum"=w301) -> ("error out"=w282:errorcluster, "refnum out"=w283:T8)  [unwired: 4 in, 1 out]
                    n110 = call-poly <vilib>:"Write Key.vi"("section"=w195, "error in (no error)"=w282, "value"=w258, "key"="aiconfigmaxv", "refnum"=w283) -> ("error out"=w267:errorcluster, "refnum out"=w268:T8)  [unwired: 4 in, 1 out]
                    n111 = call-poly <vilib>:"Write Key.vi"("section"=w195, "error in (no error)"=w267, "value"=w257, "key"="aiconfigminv", "refnum"=w268) -> ("error out"=w265:errorcluster, "refnum out"=w266:T8)  [unwired: 4 in, 1 out]
                    n112 = local read "Catch Song\nFraction"() -> (w219:dbl)
                    n113 = call-poly <vilib>:"Write Key.vi"("section"=w195, "error in (no error)"=w265, "value"=w256, "key"="aiconfigscanrate", "refnum"=w266) -> ("error out"=w223:errorcluster, "refnum out"=w225:T8)  [unwired: 4 in, 1 out]
                    n114 = local read "File State Ch"() -> (w193:i32)
                    n115 = call-poly <vilib>:"Write Key.vi"("section"=w195, "error in (no error)"=w223, "value"=w219, "key"="Catch Song", "refnum"=w225) -> ("error out"=w222:errorcluster, "refnum out"=w224:T8)  [unwired: 4 in, 1 out]
                    n116 = local read "Catch Trial\nFraction"() -> (w218:dbl)
                    n117 = local read "Syll Det Ch"() -> (w194:i32)
                    n118 = call-poly <vilib>:"Write Key.vi"("section"=w195, "error in (no error)"=w222, "value"=w218, "key"="Catch Trial", "refnum"=w224) -> ("error out"=w198:errorcluster, "refnum out"=w201:T8)  [unwired: 4 in, 1 out]
                    n119 = call-poly <vilib>:"Write Key.vi"("section"=w195, "error in (no error)"=w198, "value"=w193, "key"="FileStateChan", "refnum"=w201) -> ("error out"=w197:errorcluster, "refnum out"=w200:T8)  [unwired: 4 in, 1 out]
                    n120 = local read "Counter Rng"() -> (w281:T4)
                    n121 = local read "FFT Thresholds"() -> (w287:dbl[])
                    n122 = local read "AmpClust"() -> (w216:T1)
                    n123 = call-poly <vilib>:"Write Key.vi"("section"=w195, "error in (no error)"=w197, "value"=w194, "key"="SongInChan", "refnum"=w200) -> ("error out"=w196:errorcluster, "refnum out"=w199:T8)  [unwired: 4 in, 1 out]
                    n124 = Unbundle By Name(w216) -> ("AmpMode"=w205:u16, "Amp TH"=w204:dbl, "Max Freq(Hz)"=w203:dbl, "Min Freq(Hz)"=w202:dbl)
                    n125 = local read "FreqClust"() -> (w251:T2)
                    n126 = Array To Spreadsheet String(array=w287, 3:"%f" ("format string")) -> (spreadsheet string=w254:string)  [unwired: 1 in]
                    n127 = call "WriteCounters.vi"("Counters"=w281, "refnum"=w199) -> ("refnum out"=w217:T8)
                    n128 = call-poly <vilib>:"Write Key.vi"("section"=w228, "error in (no error)"=w196, "value"=w254, "key"="threshold", "refnum"=w217) -> ("error out"=w249:errorcluster, "refnum out"=w250:T8)  [unwired: 4 in, 1 out]
                    n129 = Unbundle By Name(w251) -> ("Min Freq(Hz)"=w240:dbl, "Max Freq(Hz)"=w239:dbl, "Freq TH Min(Hz)"=w238:dbl, "NBins"=w237:i32, "Freq TH Max(Hz)"=w236:dbl, "FreqMode"=w226:u16)
                    n130 = call-poly <vilib>:"Write Key.vi"("section"=w228, "error in (no error)"=w249, "value"=w240, "key"="Min Freq", "refnum"=w250) -> ("error out"=w248:errorcluster, "refnum out"=w244:T8)  [unwired: 4 in, 1 out]
                    n131 = call-poly <vilib>:"Write Key.vi"("section"=w228, "error in (no error)"=w248, "value"=w239, "key"="Max Freq", "refnum"=w244) -> ("error out"=w247:errorcluster, "refnum out"=w243:T8)  [unwired: 4 in, 1 out]
                    n132 = call-poly <vilib>:"Write Key.vi"("section"=w228, "error in (no error)"=w247, "value"=w238, "key"="Freq TH Min", "refnum"=w243) -> ("error out"=w246:errorcluster, "refnum out"=w242:T8)  [unwired: 4 in, 1 out]
                    n133 = call-poly <vilib>:"Write Key.vi"("section"=w228, "error in (no error)"=w246, "value"=w237, "key"="NBins", "refnum"=w242) -> ("error out"=w245:errorcluster, "refnum out"=w241:T8)  [unwired: 4 in, 1 out]
                    n134 = call-poly <vilib>:"Write Key.vi"("section"=w228, "error in (no error)"=w245, "value"=w236, "key"="Freq TH Max", "refnum"=w241) -> ("error out"=w229:errorcluster, "refnum out"=w230:T8)  [unwired: 4 in, 1 out]
                    n135 = call-poly <vilib>:"Write Key.vi"("section"=w228, "error in (no error)"=w229, "value"=w226, "key"="Freq Mode", "refnum"=w230) -> ("error out"=w211:errorcluster, "refnum out"=w215:T8)  [unwired: 4 in, 1 out]
                    n136 = call-poly <vilib>:"Write Key.vi"("section"=w190, "error in (no error)"=w211, "value"=w205, "key"="Amp Mode" ("section"), "refnum"=w215) -> ("error out"=w210:errorcluster, "refnum out"=w214:T8)  [unwired: 4 in, 1 out]
                    n137 = call-poly <vilib>:"Write Key.vi"("section"=w190, "error in (no error)"=w210, "value"=w204, "key"="Amp TH" ("section"), "refnum"=w214) -> ("error out"=w209:errorcluster, "refnum out"=w213:T8)  [unwired: 4 in, 1 out]
                    n138 = call-poly <vilib>:"Write Key.vi"("section"=w190, "error in (no error)"=w209, "value"=w203, "key"="Max Freq" ("section"), "refnum"=w213) -> ("error out"=w208:errorcluster, "refnum out"=w212:T8)  [unwired: 4 in, 1 out]
                    n139 = call-poly <vilib>:"Write Key.vi"("section"=w190, "error in (no error)"=w208, "value"=w202, "key"="Min Freq" ("section"), "refnum"=w212) -> ("error out"=w206:errorcluster, "refnum out"=w207:T8)  [unwired: 4 in, 1 out]
                    n140 = call <vilib>:"Close Config Data.vi"("error in (no error)"=w206, "refnum"=w207) -> ()  [unwired: 8 in, 2 out]
                  }
                  frame True {
                  }
                }
                n141 = property on="Load Config" class="Bool (strict)"("Disabled"=w180) -> ()  [unwired: 2 in, 2 out]
              }
            }
            n142 = local write "Save Config"(w176) -> ()
          }
          frame #2 {
          }
        }
        n143 = local read "stop"() -> (w6:bool)
        n144 = Stop(stop? (T)=w6) -> ()
        n145 = Wait (ms)(milliseconds to wait=u32 5) -> ()  [unwired: 1 out]
      }
    }
    frame #1 {
      w330 = u8 2
      # "used for Oscilloscope x-scale resizing"
      # "vvvv Read .wav File Data into 'Sound' Array vvvv"
      # "This checks if template input is a path constant,\nand if not, creates new template string of 1's?\n-SEAN"
      # "This panel (index 1) is for initialization of variables, files, and \ntemplates  -SEAN"
      n146 = local write "N Catch Esc"(i16 0 ("Esc Catch")) -> ()
      n147 = call <vilib>:"Snd Read Wave File.vi"("wave file path"="Output Sound") -> ("sound format"=→"Sound Format":T9, "mono 16-bit"=w318:i16[])  [unwired: 4 in, 5 out]
      n148 = local write "Memory Lag"(TRUE ("Memory Lag")) -> ()
      n149 = local write "First Dat"(FALSE ("First Dat")) -> ()
      n150 = local write "stop"(FALSE ("stop")) -> ()
      n151 = local write "File Open?"(FALSE ("FileOpen?")) -> ()
      n152 = local write "AO Started?"(TRUE ("AO Started?")) -> ()
      n153 = local write "Trigger"(FALSE ("Trigger")) -> ()
      n154 = local write "Too Much Data"(FALSE ("Too Much Data")) -> ()
      n155 = Absolute Value(x=w318) -> (abs(x)=w319:i16[])
      n156 = Array Max & Min(array=w319) -> (max value=w317:i16)  [unwired: 3 out]
      n157 = Divide(x=w318, y=w317) -> (x/y=w315:dbl[])
      n158 = local write "N Files"(i16 1 ("N Files")) -> ()
      n159 = local write "N Trig"(u32 0 ("N Trig")) -> ()
      n160 = Multiply(x=9.9, y=w315) -> (x*y=w316:dbl[])
      n161 = local read "Catch Song\nFraction"() -> (w349:dbl)
      n162 = Multiply(x=w316, y="AO Amp Fac") -> (x*y=→"Sound":dbl[])
      n163 = property on="Index" class="DigNum (strict)"("Visible"=FALSE) -> ()  [unwired: 2 in, 2 out]
      n164 = Random Number (0-1)() -> (number: 0 to 1=w348:dbl)
      n165 = Less Or Equal?(x=w348, y=w349) -> (x <= y?=w347:bool)
      n166 = local write "Catch Song?"(w347) -> ()
      n167 = local write "Load Config"(FALSE ("Load Config")) -> ()
      n168 = local write "Save Config"(FALSE ("Save Config")) -> ()
      n169 = property on="Load Config" class="Bool (strict)"("Disabled"=w330) -> ()  [unwired: 2 in, 2 out]
      n170 = property on="Save Config" class="Bool (strict)"("Disabled"=w330) -> ()  [unwired: 2 in, 2 out]
      n171 = Equal?(x="Templates", y=path "") -> (x = y?=w336:bool)
      n172 = property on="AO task" class="DAQmxName (strict)"("Visible"=FALSE) -> ()  [unwired: 2 in, 2 out]
      n173 = property on="Sound Rates" class="Arr (strict)"("Visible"=FALSE ("Write Attribute")) -> ()  [unwired: 2 in, 2 out]
      n174 = property on="DOtask" class="DAQmxName (strict)"("Visible"=FALSE ("Write Attribute")) -> ()  [unwired: 2 in, 2 out]
      n175 = property on="Outfile RefNum" class="Ref (strict)"("Visible"=FALSE ("Write Attribute")) -> ()  [unwired: 2 in, 2 out]
      n176 = property on="AI Actual Update" class="DigNum (strict)"("Visible"=FALSE ("Write Attribute")) -> ()  [unwired: 2 in, 2 out]
      n177 = case shown="True" w336 {
        tunnel: "Templates" -> [w383 _]
        tunnel: [w382 w391] -> w335
        frame False {
          n178 = call-poly <vilib>:"Read Delimited Spreadsheet.vi"("file path (dialog if empty)"=w383, "format (%.3f)"="%.5e", "delimiter (\\t)"=" " ("delimiter (Tab)")) -> ("new file path (Not A Path if cancelled)"=w384:path, "all rows"=w382:dbl[][])  [unwired: 7 in, 4 out]
          n179 = local write "Templates"(w384) -> ()
        }
        frame True {
          n180 = Initialize Array(0.0 ("element"), 1 ("dimension size")) -> (w389:dbl[])
          n181 = local write "FFT Thresholds"(w389) -> ()
          n182 = local write "Counter Rng"(T7 [{"Min"=0, "Max"=1, "Not"=FALSE, "Mode"=FALSE, 0, TRUE}] ("Counter Rng")) -> ()
          n183 = Initialize Array(1.0 ("element"), 128 ("dimension size"), 1 ("dimension size")) -> (w391:dbl[][])
        }
      }
      n184 = Initialize Array(0.0 ("Element Data"), 0 ("Dimension Size")) -> (w312:dbl[])
      n185 = local write "Total Data T"(0.0 ("Total Data Time")) -> ()
      n186 = local write "Manual Trigger"(FALSE ("Manual Trigger")) -> ()
      n187 = local write "Trig Times"(w312) -> ()
      n188 = local write "Temp Out"(w312) -> ()
      n189 = local write "Syll Freqs"(w312) -> ()
      n190 = local write "T snc trig"(0.0 ("T snc trig")) -> ()
      n191 = local write "N Detect"(0 ("N Detect")) -> ()
      n192 = local write "Mean"(0.0 ("Mean")) -> ()
      n193 = Array Size(array=w335) -> (size(s)=w364:i32[])
      n194 = local read "FFT Thresholds"() -> (w378:dbl[])
      n195 = local read "Counter Rng"() -> (w353:T4)
      n196 = Array Size(array=w335) -> (size(s)=w380:i32[])
      n197 = Index Array(array=w364, index=1 ("Index")) -> (element=w333:i32)
      n198 = local read "Threshold Error"() -> (w361:errorcluster)
      n199 = Bundle By Name(cluster=w361, "status"=FALSE ("Bundle Element"), "code"=0 ("Bundle Element"), "source"="" ("Bundle Element")) -> (w360:errorcluster)
      n200 = Index Array(array=w380, index=1 ("Index")) -> (element=w354:i32)
      n201 = Array Size(array=w378) -> (size(s)=w334:i32)
      n202 = Array Size(array=w353) -> (size(s)=w377:i32)
      n203 = for {
        N: w333 -> [_]
        tunnel: w335 -> [w408]
        tunnel: [w398] -> w362 mode=indexing
        i -> [w409]
        w406 = 6 ("index")
        # "Normalize the templates\nSquare here instead of \nSQRT during TAF"
        n204 = Index Array(array=w408, index (col)=w409) -> (element=w407:dbl[])  [unwired: 1 in]
        n205 = Array Subset(array=w407, index=w406) -> (w403:dbl[])  [unwired: 1 in]
        n206 = Initialize Array(0.0 ("element"), w406) -> (w404:dbl[])
        n207 = Build Array (concatenate)(w404, w403) -> (w402:dbl[])
        n208 = Array Max & Min(array=w402) -> (min value=w401:dbl)  [unwired: 3 out]
        n209 = Subtract(x=w402, y=w401) -> (x-y=w400:dbl[])
        n210 = Array Max & Min(array=w400) -> (max value=w399:dbl)  [unwired: 3 out]
        n211 = Divide(x=w400, y=w399) -> (x/y=w398:dbl[])
      }
      n212 = property on="Templates" class="Arr (strict)"("Number of Columns"=w333) -> ()  [unwired: 2 in, 2 out]
      n213 = local write "Threshold Error"(w360) -> ()
      n214 = property on="Counters" class="Arr (strict)"("Number of Rows"=w354) -> ()  [unwired: 2 in, 2 out]
      n215 = Not Equal?(x=w354, y=w334) -> (x != y?=w373:bool)
      n216 = Not Equal?(x=w354, y=w377) -> (x != y?=w372:bool)
      n217 = property on="FFT Thresholds" class="Arr (strict)"("Number of Rows"=w334) -> ()  [unwired: 2 in, 2 out]
      n218 = local read "Counter Rng"() -> (w341:T4)
      n219 = stacked-sequence {
        tunnel: w360 -> [_]
        tunnel: w373 -> [w411]
        tunnel: w372 -> [w410]
        frame #0 {
          n220 = case shown="True" w410 {
            tunnel: [w413 w414] -> w412
            frame False {
              n221 = local read "Threshold Error"() -> (w413:errorcluster)
            }
            frame True {
              n222 = local read "Threshold Error"() -> (w414:errorcluster)
              n223 = Bundle By Name(cluster=w414, "status"=TRUE ("Bundle Element"), "code"=-2 ("Bundle Element"), "source"="Counter Rng size wrong!" ("Bundle Element")) -> (w415:errorcluster)
              "Threshold Error" <- w415
              n224 = call <vilib>:"Simple Error Handler.vi"("type of dialog (OK msg:1)"=2, "error in (no error)"=w415) -> ()  [unwired: 3 in, 5 out]
            }
          }
          n225 = case shown="True" w411 {
            tunnel: w412 -> [_ w425]
            frame False {
            }
            frame True {
              n226 = Bundle By Name(cluster=w425, "status"=TRUE ("Bundle Element"), "code"=-1 ("Bundle Element"), "source"="Threshold size wrong!" ("Bundle Element")) -> (w420:errorcluster)
              n227 = local write "Threshold Error"(w420) -> ()
              n228 = call <vilib>:"Simple Error Handler.vi"("type of dialog (OK msg:1)"=2, "error in (no error)"=w420) -> ()  [unwired: 3 in, 5 out]
            }
          }
        }
      }
      n229 = for {
        tunnel: w341 -> [w397] mode=indexing
        tunnel: [w395] -> w340 mode=indexing
        n230 = Unbundle By Name(w397) -> ("Max"=w396:i16)
        n231 = Increment(x=w396) -> (x+1=w395:i16)
      }
      "Counters" <- w340
      n232 = Transpose 2D Array(2D array=w362) -> (transposed array=w329:dbl[][])
      "Templates" <- w329
      n233 = Array Size(array=w329) -> (size(s)=w328:i32[])
      n234 = Index Array(array=w328, index=0) -> (element=w327:i32)
      n235 = Multiply(x=w327, y=2) -> (x*y=→"NFFT":i32)
      "Index" <- 0 ("Index")
    }
    frame #2 {
      w441 = -1 items=["Default"=-1, "RSE"=10083, "NRSE"=10078, "Differential"=10106, "Pseudodifferential"=12529] ("input terminal configuration")
      w442 = 10083 items=["Default"=-1, "RSE"=10083, "Differential"=10106, "Pseudodifferential"=12529] ("output terminal configuration")
      w453 = 0 ("dimension size")
      w454 = i16 0 ("element")
      w475 = 10178 items=["Finite Samples"=10178, "Continuous Samples"=10123, "Hardware Timed Single Point"=12522] ("sample mode")
      w519 = 10123 items=["Finite Samples"=10178, "Continuous Samples"=10123, "Hardware Timed Single Point"=12522] ("sample mode")
      # "<<-----------------\nThis section runs in parallel with the main loop to allow listening to the specified UDP port. It will set the global trigger variable when a UDP packet is received \n<<-----------------"
      # "vvvv Initialization for Oscilloscope vvvv"
      # "^^^CONFIGURE DIGITAL TRIGGER TASK ^^^"
      # "^^^ CONFIGURE AUDIO INPUT TASK ^^^"
      # "vvv CONFIGURE AUDIO OUTPUT TASK vvv"
      n236 = UDP Open(11:"UDP_port") -> (port=w428:refnum<k16>, 0:w429:errorcluster)  [unwired: 4 in, 1 out]
      n237 = while {
        tunnel: [w546] -> w432
        tunnel: [w545] -> w431
        tunnel: w429 -> [w544]
        tunnel: w428 -> [w543]
        tunnel: "occurrence" -> [w539]
        stop <- FALSE stop-if-true
        # "this loop waits here, listening on the specified port until a message is received, then it passes into the structure to the right to set the local trigger variable"
        n238 = UDP Read(connection ID=w543, timeout ms (25000)=-1, 8:w544) -> (data out=w541:string, error out=w546:errorcluster, 3:w545:refnum<k16>)  [unwired: 1 in, 2 out]
        "UDP_packet_contents" <- w541
        n239 = case shown="No Error" w546 {
          tunnel: w541 -> [w556 _]
          tunnel: w539 -> [w547 _]
          frame No Error {
            n240 = flat-sequence {
              tunnel: w547 -> [w558]
              frame #0 {
                "UDP Trig" <- TRUE
              }
              frame #1 {
                n241 = Wait on Occurrence(2:w558) -> ()  [unwired: 2 in, 1 out]
              }
              frame #2 {
                n242 = local write "UDP Trig"(FALSE) -> ()
              }
            }
            n243 = Fract/Exp String To Number(string=w556) -> (number=w550:dbl)  [unwired: 3 in, 1 out]
            n244 = Get Date/Time In Seconds() -> (seconds since 1Jan1904=w554:timestamp)
            n245 = To Double Precision Float(number=w554) -> (double precision float=w548:dbl)
            "packet_timestamp_sec" <- w548
            n246 = Add(x=w550, y=2082844800.0) -> (x+y=w549:dbl)
            "time_when_received_sec" <- w549
            n247 = Subtract(x=w548, y=w549) -> (x-y=w555:dbl)
            n248 = Multiply(x=w555, y=1000.0) -> (x*y=→"packet_latency_ms":dbl)
          }
          frame Error {
            n249 = Stop() -> ()  [unwired: 1 in]
          }
        }
      }
      n250 = Unbundle By Name("Analog Output Config") -> ("Min Voltage"=w508:i8, "Max Voltage"=w507:u16)  [unwired: 2 out]
      n251 = local read "Sound"() -> (w493:dbl[])
      n252 = local read "Data Bef Trig(s)"() -> (w518:dbl)
      n253 = Build Array("TAF Trig Out", "REC Trig Pin", "REC LED Pin") -> (w435:tag[])
      n254 = Unbundle By Name("Analog Input Config") -> ("Min Voltage"=w526:i8, "Max Voltage"=w525:i8, "AI Channels"=w524:string, "Chan Name"=w523:string, "Scan Rate(kHz)"=w521:dbl)
      "Max Voltage" <- w525
      n255 = Array Size(array=w493) -> (size(s)=w474:i32)
      n256 = local read "Sound Format"() -> (w528:T3)
      n257 = call-poly <vilib>:"DAQmx Create Virtual Channel.vi"("maximum value"=w507, "minimum value"=w508, "output terminal configuration"=w442, "physical channels"=tag "Dev1/ao0") -> ("task out"=w506:refnum<k21>, "error out"=w503:errorcluster)  [unwired: 10 in]
      n258 = call <vilib>:"DAQmx Flatten Channel String.vi"("names in"=w435) -> ("names out"=w436:string)  [unwired: 13 in, 1 out]
      n259 = Multiply(x=2, y=w474) -> (x*y=w504:i32)
      n260 = Multiply(x=w521, y=1000.0) -> (x*y=w515:dbl)
      n261 = Multiply(x=w518, y=2) -> (x*y=w516:dbl)
      n262 = call <vilib>:"DAQmx Configure Output Buffer.vi"("task/channels in"=w506, "buffer size (in samples per channel)"=w504, "error in"=w503) -> ("task out"=w502:refnum<k21>, "error out"=w500:errorcluster)  [unwired: 11 in]
      n263 = Multiply(x=w515, y=w516) -> (x*y=w514:dbl)
      n264 = Unbundle By Name(w528) -> ("Rate"=w534:u16)
      n265 = Round Toward +Infinity(x=w514) -> (ceil(x): smallest int >= x=w513:dbl)
      n266 = Index Array(array="Sound Rates", index=w534) -> (element=w501:dbl)
      n267 = call-poly <vilib>:"DAQmx Create Virtual Channel.vi"("lines"=w436, "line grouping"=0) -> ("task out"=w460:refnum<k21>, "error out"=w483:errorcluster)  [unwired: 12 in]
      n268 = To Long Integer(number=w513) -> (32bit integer=w512:i32)
      "Buffer Size" <- w512
      n269 = local read "Analog Output Config"() -> (w498:T6)
      n270 = call-poly <vilib>:"DAQmx Timing.vi"("task/channels in"=w502, "sample mode"=w475, "samples per channel"=w474, "rate"=w501, "error in"=w500) -> ("task out"=w499:refnum<k21>, "error out"=w496:errorcluster)  [unwired: 9 in]
      n271 = Unbundle By Name(w498) -> ("TAF Trig In"=w497:tag)
      n272 = call <vilib>:"DAQmx Start Task.vi"("task/channels in"=w460, "error in"=w483) -> ("task out"=w482:refnum<k21>, "error out"=w481:errorcluster)  [unwired: 12 in]
      n273 = call-poly <vilib>:"DAQmx Trigger.vi"("task/channels in"=w499, "source"=w497, "error in"=w496) -> ("task out"=w495:refnum<k21>, "error out"=w494:errorcluster)  [unwired: 11 in]
      n274 = call-poly <vilib>:"DAQmx Write.vi"("task/channels in"=w482, "data"=bool[] [FALSE, FALSE, FALSE], "error in"=w481) -> ("task out"=→"DOtask":refnum<k21>, "error out"=w468:errorcluster)  [unwired: 10 in, 1 out]
      n275 = call-poly <vilib>:"DAQmx Write.vi"("task/channels in"=w495, "data"=w493, "error in"=w494) -> ("task out"=w492:refnum<k21>, "number of samples written per channel"=→"AO Nwrtn":u32, "error out"=w491:errorcluster)  [unwired: 10 in]
      n276 = call <vilib>:"DAQmx Start Task.vi"("task/channels in"=w492, "error in"=w491) -> ("task out"=w488:refnum<k21>, "error out"=w473:errorcluster)  [unwired: 12 in]
      "AO task" <- w488
      n277 = call-poly <vilib>:"DAQmx Create Virtual Channel.vi"("maximum value"=w525, "minimum value"=w526, "input terminal configuration"=w441, "physical channels"=w524, "name to assign"=w523, "error in"=w473) -> ("task out"=w522:refnum<k21>, "error out"=w511:errorcluster)  [unwired: 8 in]
      n278 = call-poly <vilib>:"DAQmx Timing.vi"("task/channels in"=w522, "sample mode"=w519, "samples per channel"=w512, "rate"=w515, "source"="Clock Source", "error in"=w511) -> ("task out"=w472:refnum<k21>, "error out"=w470:errorcluster)  [unwired: 8 in]
      n279 = property class="DAQmx Read"(reference=w472) -> ("Advanced:Number of Channels"=w477:u32)  [unwired: 1 in, 2 out]
      "N AI Chan" <- w477
      n280 = property class="DAQmx Timing"(reference=w472) -> ("Sample Clock:Rate"=w458:dbl)  [unwired: 1 in, 2 out]
      "AI Rate" <- w458
      n281 = Multiply(x=w458, y="Data Bef Trig(s)") -> (x*y=w538:dbl)
      n282 = Reciprocal(x=w458) -> (1/x=w461:dbl)
      "AI Actual Update" <- w461
      n283 = Round Toward +Infinity(x=w538) -> (ceil(x): smallest int >= x=w537:dbl)
      n284 = UDP Close(connection ID=w431, 8:w432) -> (error out=→"UDP Packet Error":errorcluster)  [unwired: 1 out]
      n285 = local read "AI Rate"() -> (w450:dbl)
      n286 = To Long Integer(number=w537) -> (32bit integer=w462:i32)
      "DataBefTrig" <- w462
      n287 = local write "AO Error"(w473) -> ()
      n288 = local read "NFFT"() -> (w459:i32)
      n289 = Initialize Array(i16 0 ("Element Data"), w477, w462) -> (w456:i16[][])
      n290 = property class="DAQmx Timing"(reference=w488) -> ("Sample Clock:Rate"=w487:dbl)  [unwired: 1 in, 2 out]
      "Real AO Rate" <- w487
      n291 = Multiply(x=2.0, y=w450) -> (x*y=w446:dbl)
      n292 = Initialize Array(i16 0 ("element"), w446) -> (w445:i16[])
      n293 = stacked-sequence {
        tunnel: w472 -> [w565]
        tunnel: [w565] -> w471
        tunnel: w470 -> [w564]
        tunnel: [w564] -> w469
        tunnel: w456 -> [_]
        tunnel: w468 -> [_]
        tunnel: w459 -> [w563]
        tunnel: w458 -> [w562]
        tunnel: [w561] -> w457
        frame #0 {
          n294 = call "get_freqvals.vi"("Fsample"=w562, "NFFT"=w563) -> ("FreqVals"=w561:dbl[])
        }
      }
      "FreqVals" <- w457
      n295 = Divide(x=w487, y=w474) -> (x/y=w465:dbl)
      n296 = To Double Precision Float(number=w445) -> (double precision float=w444:dbl[])
      n297 = local read "Data Aft Trig(s)"() -> (w533:dbl)
      n298 = local write "Prev Spike"(w445) -> ()
      n299 = Multiply(x=w465, y=1.01) -> (x*y=w451:dbl)
      "AO Len" <- w451
      n300 = case shown="True" "Auto Trig Refrac?" {
        tunnel: w451 -> [_ w560]
        frame False {
        }
        frame True {
          n301 = local write "Trig Refrac(s)"(w560) -> ()
        }
      }
      n302 = Multiply(x=w461, y=w462) -> (x*y=→"T Bef":dbl)
      n303 = property on="Neural Data" class="WFChart (strict)"("History Data"=w444) -> (error out=w443:errorcluster)  [unwired: 2 in, 1 out]
      n304 = property on="Neural Data" class="WFChart (strict)"(error in=w443, "XScale.Maximum"=w446, "XScale.Minimum"=0.0 ("X Scale.Range:Minimum")) -> ()  [unwired: 1 in, 2 out]
      n305 = call <vilib>:"DAQmx Start Task.vi"("task/channels in"=w471, "error in"=w469) -> ("task out"=w466:refnum<k21>, "error out"=w467:errorcluster)  [unwired: 12 in]
      n306 = Increment(x=w533) -> (x+1=w532:dbl)
      n307 = Initialize Array(w454, w453) -> (w455:i16[])
      n308 = Initialize Array(w454, w453) -> (w535:i16[])
      n309 = while {
        shift-left: 0 -> [w627]
        shift-right: [w626] -> _
        shift-left: w535 -> [w631]
        shift-right: [w630] -> _
        shift-left: w532 -> [w604]
        shift-right: [w632] -> _
        tunnel: w461 -> [_]
        shift-left: w456 -> [w614]
        shift-right: [w582] -> _
        tunnel: w467 -> [w621]
        tunnel: [w619] -> w510
        tunnel: [w620] -> w478
        tunnel: w488 -> [_]
        tunnel: [w618] -> w486
        tunnel: [w617] -> w485
        tunnel: [w616] -> w479
        tunnel: w466 -> [w615]
        shift-right: [w588] -> _
        shift-left: w455 -> [w589]
        shift-right: [w575] -> _
        shift-left: _ -> [w574]
        tunnel: "occurrence" -> [w566]
        stop <- w607 continue-if-true
        # "This block computes timing and \nsends TTL pulses to control the\nCamera REC and the Sync LED"
        # "Circular Buffer"
        # "^^^This Structure Computes the Oscilloscope Style Edge Triggering^^^"
        # "current data"
        # "buffer data"
        n310 = call-poly <vilib>:"DAQmx Read.vi"("task/channels in"=w615, "timeout"=0.0, "error in"=w621) -> ("task out"=w620:refnum<k21>, "data"=w583:i16[][], "error out"=w619:errorcluster)  [unwired: 10 in]
        "AI Error" <- w619
        n311 = Increment(x="WhichChan") -> (x+1=w581:i32)
        n312 = local read "N AI Chan"() -> (w580:i32)
        n313 = Greater Or Equal?(x=w580, y=w581) -> (x >= y?=w577:bool)
        n314 = call "PullOutData.vi"("WhichInd"="Syll Det Ch", "InputArray"=w583) -> ("OutVec"=w591:i16[])
        n315 = And(x="Plot2", y=w577) -> (x .and. y?=w576:bool)
        n316 = Array Size(array=w591) -> (size(s)=→"N Read":i32)
        n317 = local read "Index"() -> (w613:i32)
        n318 = Not Equal?(x="Amp Det Ch", y="Syll Det Ch") -> (x != y?=w593:bool)
        n319 = case shown="False" "Time Test?" {
          tunnel: w583 -> [_ w658]
          frame False {
          }
          frame True {
            n320 = Index Array(array=w658, index (row)=0) -> (element=w656:i16[])  [unwired: 1 in]
            n321 = Array Max & Min(array=w656) -> (max value=w655:i16)  [unwired: 3 out]
            n322 = Greater?(x=w655, y=i16 500) -> (0:w653:bool)
            n323 = case shown="True" w653 {
              frame False {
              }
              frame True {
                n324 = local read "Trig Time"() -> (w660:u32)
                n325 = Tick Count (ms)() -> (millisecond timer value=w661:u32)
                n326 = Subtract(x=w661, y=w660) -> (x-y=→"Read dt":u32)
              }
            }
          }
        }
        n327 = call "arrayshift_I16.vi"("NewArray"=w583, "IndexIn"=w613, "SaveArray"=w614) -> ("Too Big"=→"Too Much Data":bool, "IndexOut"=w584:i32, "OutArray"=w582:i16[][])
        n328 = case shown="True" w576 {
          tunnel: w584 -> [_ w675]
          tunnel: w583 -> [_ w674]
          tunnel: w582 -> [_ w673]
          tunnel: "WhichChan" -> [_ w670]
          tunnel: [w666 w668] -> w575
          tunnel: w574 -> [w666 w667]
          frame False {
          }
          frame True {
            # "This structure only plots a waveform if it crosses the height threshold while inside a band of possible indexes near the middle of the plot window. This gives the illusion that the spike remain still in time. Since this is checked every loop, with a smoothly running buffer, virtually no spikes should be lost"
            n329 = local read "AI Rate"() -> (w669:dbl)
            n330 = local read "Max Voltage"() -> (w671:dbl)
            n331 = case shown="True" "Trig Edge?" {
              selector: "Trig Edge?" -> [w679 w718]
              tunnel: w675 -> [_ w724]
              tunnel: w670 -> [w682 w726]
              tunnel: w674 -> [w681 _]
              tunnel: [w680 w719] -> w672
              tunnel: w673 -> [_ w727]
              tunnel: w671 -> [_ w715]
              tunnel: w669 -> [_ w699]
              tunnel: [w678 w697] -> w668
              tunnel: w667 -> [w678 w696]
              frame False {
                # "^^^This box zooms all the way out in time (x-axis) to include all^^^\n        of the points available in the chart history. This actually can be\n        a memory-heavy task, so we only compute once at the\n        beginning, thanks to Memory Lag, which\n        contains a bit value indicating a recent switch in mode. There\n        is a corresponding section in the False of this structure to zoom into\n        the size of the user-defined time-window."
                n332 = flat-sequence {
                  tunnel: w679 -> [w689]
                  frame #0 {
                    n333 = local read "Memory Lag"() -> (w683:bool)
                    n334 = case shown="True" w683 {
                      frame False {
                      }
                      frame True {
                        n335 = property on="Neural Data" class="WFChart (strict)"() -> ("History Data"=w688:sgl[])  [unwired: 2 in, 2 out]
                        n336 = Array Size(array=w688) -> (size(s)=w687:i32)
                        n337 = Decrement(x=w687) -> (x-1=w686:i32)
                        n338 = To Double Precision Float(number=w686) -> (double precision float=w685:dbl)
                        n339 = property on="Neural Data" class="WFChart (strict)"("XScale.Maximum"=w685, "XScale.Minimum"=0.0 ("X Scale.Range:Minimum")) -> ()  [unwired: 2 in, 2 out]
                      }
                    }
                  }
                  frame #1 {
                    "Memory Lag" <- w689
                  }
                }
                n340 = Index Array(array=w681, index (row)=w682) -> (element=w680:i16[])  [unwired: 1 in]
              }
              frame True {
                # "This creates a Window\nsized buffer"
                # "100mV\nband \nthreshold"
                n341 = flat-sequence {
                  tunnel: w716 -> [w740]
                  tunnel: "Window (ms)" -> [w736]
                  tunnel: [w736] -> w697
                  tunnel: w696 -> [w735]
                  tunnel: w718 -> [w748]
                  frame #0 {
                    # "Window\nChange?"
                    n342 = local read "Memory Lag"() -> (w739:bool)
                    n343 = Not Equal?(x=w736, y=w735) -> (x != y?=w734:bool)
                    n344 = First Call?() -> (First Call?: T/F=w732:bool)
                    n345 = Not(x=w739) -> (.not. x?=w737:bool)
                    n346 = Or(x=w734, y=w732) -> (x .or. y?=w733:bool)
                    n347 = Or(x=w737, y=w733) -> (x .or. y?=w738:bool)
                    n348 = case shown="True" w738 {
                      tunnel: w740 -> [_ w742]
                      frame False {
                      }
                      frame True {
                        n349 = property on="Neural Data" class="WFChart (strict)"() -> ("History Data"=w747:sgl[])  [unwired: 2 in, 2 out]
                        n350 = Decrement(x=w742) -> (x-1=w741:u16)
                        n351 = Array Size(array=w747) -> (size(s)=w746:i32)
                        n352 = Decrement(x=w746) -> (x-1=w745:i32)
                        n353 = To Double Precision Float(number=w745) -> (double precision float=w743:dbl)
                        n354 = Subtract(x=w743, y=w741) -> (x-y=w744:dbl)
                        n355 = property on="Neural Data" class="WFChart (strict)"("XScale.Maximum"=w743, "XScale.Minimum"=w744) -> ()  [unwired: 2 in, 2 out]
                      }
                    }
                  }
                  frame #1 {
                    n356 = local write "Memory Lag"(w748) -> ()
                  }
                }
                n357 = Decrement(x=w724) -> (x-1=w723:i32)
                n358 = Index Array(array=w727, index (row)=w726) -> (element=w725:i16[])  [unwired: 1 in]
                n359 = Divide(x=w699, y=1000.0) -> (x/y=w730:dbl)
                n360 = To Unsigned Word Integer(number=w730) -> (unsigned 16bit integer=w717:u16)
                n361 = Multiply(x="Window (ms)", y=w717) -> (x*y=w716:u16)
                n362 = Subtract(x=w724, y=w716) -> (x-y=w728:i32)
                n363 = Greater Or Equal To 0?(x=w728) -> (x >= 0?=w731:bool)
                n364 = local read "DataBefTrig"() -> (w722:i32)
                n365 = Divide(x=w716, y=u16 2) -> (x/y=w707:sgl)
                n366 = Round Toward -Infinity(1:w707) -> (0:w706:sgl)
                n367 = Divide(x=w706, y=i16 10) -> (x/y=w709:sgl)
                n368 = Decrement(x=w722) -> (x-1=w721:i32)
                n369 = case shown="False" w731 {
                  tunnel: w728 -> [w759 w763]
                  tunnel: w716 -> [_ w761]
                  tunnel: w725 -> [w758 w762]
                  tunnel: [w753 w760] -> w704
                  tunnel: w723 -> [w752 _]
                  tunnel: w721 -> [w751 _]
                  frame False {
                    n370 = Array Subset(array=w758, index=0, length=w752) -> (w755:i16[])
                    n371 = Add(x=w751, y=w759) -> (x+y=w757:i32)
                    n372 = Array Subset(array=w758, index=w757) -> (w756:i16[])  [unwired: 1 in]
                    n373 = Build Array (concatenate)(w756, w755) -> (w753:i16[])
                  }
                  frame True {
                    n374 = Array Subset(array=w762, index=w763, length=w761) -> (w760:i16[])
                  }
                }
                n375 = Decrement(x=w706) -> (x-1=w711:sgl)
                n376 = Round Toward +Infinity(x=w709) -> (ceil(x): smallest int >= x=w708:sgl)
                n377 = Array Subset(array=w704, index=w711, length=w708) -> (w700:i16[])
                n378 = Add(x=sgl 100.0, y="Threshold (mV)") -> (x+y=w692:sgl)
                n379 = call-poly <vilib>:"Mean.vi"("X"=w700) -> ("mean"=w693:dbl)  [unwired: 1 out]
                n380 = call "NetSlopeDetect.vi"("SigInput"=w700, "+/- Slope"="Slope Trig", "On/Off"=TRUE) -> ("Boolean"=w705:bool)  [unwired: 8 in]
                n381 = To Word Integer(number=w693) -> (16bit integer=w714:i16)
                n382 = call "Int16Scale_mV_1Elem.vi"("Max Voltage"=w715, "Int16Elem"=w714) -> ("Scaled mV Elem"=w695:sgl)
                n383 = Greater Or Equal?(x=w695, y="Threshold (mV)") -> (x >= y?=w713:bool)
                n384 = Greater?(x=w692, y=w695) -> (0:w694:bool)
                n385 = And(x=w694, y=w713) -> (x .and. y?=w712:bool)
                n386 = And(x=w712, y=w705) -> (x .and. y?=w701:bool)
                n387 = case shown="True" w701 {
                  tunnel: w704 -> [_ w750]
                  tunnel: [w749 w750] -> w719
                  tunnel: w701 -> [_ _]
                  frame False {
                    n388 = local read "Prev Spike"() -> (w749:i16[])
                  }
                  frame True {
                    "Prev Spike" <- w750
                  }
                }
              }
            }
            n389 = call "Int16Scale_mV_1DArray.vi"("Max Voltage"=w671, "Int16Array"=w672) -> ("Scaled mV Array"=→"Neural Data":sgl[])
          }
        }
        n390 = local write "Index"(w584) -> ()
        n391 = case shown="True" w593 {
          tunnel: [w662 w665] -> w590
          tunnel: "Amp Det Ch" -> [_ w663]
          tunnel: w583 -> [_ w664]
          tunnel: w591 -> [w662 _]
          frame False {
          }
          frame True {
            n392 = call "PullOutData.vi"("WhichInd"=w663, "InputArray"=w664) -> ("OutVec"=w665:i16[])
          }
        }
        n393 = local read "Mean"() -> (w597:dbl)
        n394 = call "TH_crossing.vi"("NewData"=w583, "Threshold"="Raw Threshold", "FileMonChan"="File State Ch", "MeanIn"=w597, "MeanSmoothFac"="Smth Fac") -> ("Crossing?"=w596:bool, "MeanOut"=→"Mean":dbl)
        n395 = case shown="True" "Plot" {
          tunnel: w591 -> [_ w764]
          frame False {
          }
          frame True {
            "Song Data" <- w764
          }
        }
        n396 = local read "Manual Trigger"() -> (w606:bool)
        n397 = local read "AO Len"() -> (w586:dbl)
        n398 = Array Size(array=w583) -> (size(s)=w629:i32[])
        n399 = Greater?(x="Data Aft Trig(s)", y=w604) -> (0:w633:bool)
        n400 = Index Array(array=w629, index=1 ("Index")) -> (element=w602:i32)
        n401 = local read "AI Actual Update"() -> (w623:dbl)
        n402 = local read "UDP Trig"() -> (w567:bool)
        n403 = Or(x=w596, y=w633) -> (x .or. y?=w610:bool)
        n404 = Negate(x=w586) -> (-x=w585:dbl)
        n405 = Not(x=w606) -> (.not. x?=w605:bool)
        n406 = Or(x=w610, y=w606) -> (x .or. y?=w569:bool)
        n407 = Multiply(x=w623, y=w602) -> (x*y=w573:dbl)
        n408 = Select(t=w604, s=w605, f=w585) -> (s? t:f=w603:dbl)
        n409 = Or(x=w567, y=w569) -> (x .or. y?=w568:bool)
        n410 = local read "AO Error"() -> (w617:errorcluster)
        n411 = local read "AO task"() -> (w618:refnum<k21>)
        n412 = Not(x="stop") -> (.not. x?=w608:bool)
        n413 = And(x=w608, y=w568) -> (x .and. y?=w570:bool)
        n414 = feedback-in #1(w570) -> ()
        n415 = feedback #1(w570) -> (w571:bool)
        n416 = Exclusive Or(1:w571, 2:w570) -> (0:w572:bool)
        n417 = case shown="False" w572 {
          tunnel: w570 -> [w634 _]
          frame False {
            n418 = call <vilib>:"High Resolution Relative Seconds.vi"() -> ("relative seconds"=w639:dbl)
            n419 = local read "tic"() -> (w638:dbl)
            n420 = Subtract(x=w639, y=w638) -> (x-y=w637:dbl)
            n421 = Greater Or Equal?(x=w637, y=0.01) -> (x >= y?=w635:bool)
            n422 = case shown="True" w635 {
              tunnel: w634 -> [_ w642]
              frame False {
              }
              frame True {
                n423 = local read "DOtask"() -> (w645:refnum<k21>)
                n424 = Build Array (concatenate)(bool[] [FALSE, FALSE] ("data"), w642) -> (w640:bool[])
                n425 = Array Subset(array=w640, index=1) -> (w643:bool[])  [unwired: 1 in]
                n426 = local write "RecSigs"(w643) -> ()
                n427 = call-poly <vilib>:"DAQmx Write.vi"("task/channels in"=w645, "data"=w640) -> ()  [unwired: 11 in, 3 out]
              }
            }
          }
          frame True {
            n428 = Build Array (concatenate)(bool[] [FALSE, TRUE] ("data"), FALSE) -> (w648:bool[])
            n429 = local read "DOtask"() -> (w652:refnum<k21>)
            n430 = call-poly <vilib>:"DAQmx Write.vi"("task/channels in"=w652, "data"=w648) -> ()  [unwired: 11 in, 3 out]
            n431 = call <vilib>:"High Resolution Relative Seconds.vi"() -> ("relative seconds"=→"tic":dbl)
            n432 = Array Subset(array=w648, index=1) -> (→"RecSigs":bool[])  [unwired: 1 in]
          }
        }
        n433 = case shown="True" w570 {
          tunnel: [w789 w838] -> w632
          tunnel: w631 -> [_ w890]
          tunnel: [w769 w843] -> w630
          tunnel: w596 -> [_ w889]
          tunnel: w603 -> [_ w888]
          tunnel: w582 -> [_ w885]
          tunnel: w583 -> [_ w884]
          tunnel: w573 -> [w773 w863]
          tunnel: w591 -> [_ w877]
          tunnel: w627 -> [w786 w880]
          tunnel: [0 w879] -> w626
          tunnel: w584 -> [_ w865]
          tunnel: [0.0 w860] -> w611
          tunnel: w608 -> [w771 w859]
          tunnel: [w770 w859] -> w607
          tunnel: w590 -> [_ w845]
          tunnel: w589 -> [_ w846]
          tunnel: [w768 w842] -> w588
          tunnel: w567 -> [_ w835]
          tunnel: w566 -> [_ w834]
          frame False {
            w765 = 0 ("dimension size")
            w766 = i16 0 ("element")
            n434 = local read "Total Data T"() -> (w781:dbl)
            n435 = local read "File Open?"() -> (w779:bool)
            n436 = local read "T snc trig"() -> (w772:dbl)
            n437 = Add(x=w773, y=w772) -> (x+y=w780:dbl)
            n438 = local write "T snc trig"(w780) -> ()
            n439 = local write "First Dat"(TRUE ("First Dat")) -> ()
            n440 = Initialize Array(0, 0) -> (w775:i32[])
            n441 = Initialize Array(0.0 ("Element Data"), 0 ("Dimension Size")) -> (w783:dbl[])
            n442 = case shown="True" w779 {
              tunnel: w781 -> [_ w808]
              tunnel: w786 -> [_ w813]
              tunnel: w783 -> [w792 w812]
              tunnel: [w792 w812] -> w767
              tunnel: w775 -> [w791 w807]
              tunnel: [w791 w807] -> w774
              tunnel: w771 -> [w790 w803]
              tunnel: [w790 w803] -> w770
              frame False {
              }
              frame True {
                w794 = FALSE ("FileOpen?")
                n443 = local read "RecSigs"() -> (w793:bool[])
                n444 = local read "Trig Times"() -> (w802:dbl[])
                n445 = local read "Outfile RefNum"() -> (w810:refnum<file>)
                n446 = local read "DOtask"() -> (w796:refnum<k21>)
                n447 = local write "File Open?"(w794) -> ()
                n448 = Greater Or Equal?(x=w808, y="Min Data Time") -> (x >= y?=w801:bool)
                n449 = Close File(refnum=w810) -> (path=w797:path, error out=w814:errorcluster)  [unwired: 1 in]
                n450 = Array Size(array=w802) -> (size(s)=w799:i32)
                n451 = Build Array (concatenate)(w794, w793) -> (w795:bool[])
                n452 = call-poly <vilib>:"DAQmx Write.vi"("task/channels in"=w796, "data"=w795) -> ()  [unwired: 11 in, 3 out]
                n453 = Greater Than 0?(x=w799) -> (x > 0?=w798:bool)
                n454 = Or(x=w798, y=w801) -> (x .or. y?=w800:bool)
                n455 = Random Number (0-1)() -> (number: 0 to 1=w805:dbl)
                n456 = Less Or Equal?(x=w805, y="Catch Song\nFraction") -> (x <= y?=w804:bool)
                n457 = case shown="True" w800 {
                  tunnel: w814 -> [w817 _]
                  tunnel: w797 -> [w816 w828]
                  tunnel: w813 -> [_ w819]
                  tunnel: [w815 w821] -> w809
                  tunnel: w808 -> [_ w823]
                  tunnel: w804 -> [w815 w821]
                  frame False {
                    n458 = Delete(path (use dialog)=w816, error in=w817) -> ()  [unwired: 3 in, 3 out]
                  }
                  frame True {
                    n459 = local read "Trig Times"() -> (w829:dbl[])
                    n460 = local read "Data Bef Trig(s)"() -> (w827:dbl)
                    n461 = local read "FFT Thresholds"() -> (w825:dbl[])
                    n462 = local read "Data Aft Trig(s)"() -> (w826:dbl)
                    n463 = local read "AI Rate"() -> (w830:dbl)
                    n464 = local read "Catch Song?"() -> (w832:bool)
                    n465 = call "WrtTempFile.vi"("Trigger Times"="Temp Out", "Input Path"=w828) -> ()  [unwired: 3 in]
                    n466 = local read "Output Sound"() -> (w820:path)
                    n467 = local read "N AI Chan"() -> (w831:i32)
                    n468 = Bundle("Data Bef Trig(s)"=w827, "Data Aft Trig(s)"=w826, "FFT Thresholds"=w825, "Output Sound"=w820) -> (w824:T10)  [unwired: 1 in]
                    n469 = local read "Syll Freqs"() -> (w818:dbl[])
                    n470 = local read "Catch?"() -> (w822:i32[])
                    n471 = call "WrtRecFile.vi"("Syll Freqs"=w818, 1:"Catch"=w822, "Samples"=w819, "N Channel"=w831, "File Info"=w824, 5:"Catch"=w832, "AI Rate"=w830, "Total Data Time"=w823, "Trigger Times"=w829, "Input Path"=w828) -> ()
                  }
                }
                "Catch Song?" <- w809
              }
            }
            n472 = local write "Trig Times"(w767) -> ()
            n473 = local write "Syll Freqs"(w767) -> ()
            n474 = local write "Temp Out"(w767) -> ()
            n475 = local write "Catch?"(w774) -> ()
            n476 = local read "Data Aft Trig(s)"() -> (w782:dbl)
            n477 = Initialize Array(w766, w765) -> (w768:i16[])
            n478 = Initialize Array(w766, w765) -> (w769:i16[])
            n479 = Increment(x=w782) -> (x+1=w789:dbl)
          }
          frame True {
            # "this part computes silence time\nby cumsumming #pts*1/32000"
            # "Triggered? (T/F)"
            # "This Part Writes the Data File"
            n480 = local read "Templates"() -> (w869:sgl[][])
            n481 = case shown="False" w889 {
              tunnel: [w944 0.0] -> w838
              tunnel: w888 -> [w945 _]
              tunnel: w863 -> [w943 _]
              frame False {
                n482 = Add(x=w945, y=w943) -> (x+y=w944:dbl)
              }
              frame True {
              }
            }
            n483 = Build Array (concatenate)(w890, w877) -> (w886:i16[])
            n484 = local read "T snc trig"() -> (w847:dbl)
            n485 = local read "Counters"() -> (w872:u32[])
            n486 = local read "T snc trig"() -> (w874:dbl)
            n487 = Build Array (concatenate)(w846, w845) -> (w844:i16[])
            n488 = local read "First Dat"() -> (w864:bool)
            n489 = Greater?(x=w874, y="Trig Refrac(s)") -> (0:w883:bool)
            n490 = case shown="False" w864 {
              tunnel: w885 -> [_ w908]
              tunnel: w884 -> [w893 _]
              tunnel: [w895 w910] -> w868
              tunnel: w865 -> [_ w907]
              frame False {
                # "Stream current data"
                n491 = local read "Output Path"() -> (w906:path)
                n492 = local read "File Open?"() -> (w898:bool)
                n493 = local read "Outfile RefNum"() -> (w899:refnum<file>)
                n494 = local read "Bird Name"() -> (w900:string)
                n495 = local read "N Files"() -> (w901:i16)
                n496 = Array Size(array=w893) -> (size(s)=w897:i32[])
                n497 = Transpose 2D Array(2D array=w893) -> (transposed array=w896:i16[][])
                n498 = Multiply Array Elements(1:w897) -> (0:w892:i32)
                n499 = Reshape Array(w896, w892) -> (w894:i16[])
                n500 = call "write_data.vi"("Data"=w894, "Root Path"=w906, "N Files In"=w901, "Bird Name"=w900, "RefNum In"=w899, "File Open In"=w898) -> ("N Files Out"=w902:i16, "File Open Out"=w903:bool, "Output File Path"=w904:path, "RefNum Out"=w905:refnum<file>)
                n501 = Array Size(array=w894) -> (size(s)=w895:i32)
                n502 = local write "Outfile RefNum"(w905) -> ()
                n503 = local write "Current File"(w904) -> ()
                n504 = local write "File Open?"(w903) -> ()
                n505 = local write "N Files"(w902) -> ()
              }
              frame True {
                # "Write out the buffer"
                n506 = for {
                  N: 2 -> [_]
                  shift-right: [w922] -> w910
                  shift-left: 0 -> [w920]
                  tunnel: w908 -> [w917]
                  tunnel: w907 -> [w916]
                  i -> [w919]
                  n507 = local read "Outfile RefNum"() -> (w929:refnum<file>)
                  n508 = local read "N Files"() -> (w932:i16)
                  n509 = Equal To 0?(x=w919) -> (x = 0?=w918:bool)
                  n510 = case shown="False" w918 {
                    tunnel: w917 -> [w938 w942]
                    tunnel: w916 -> [w935 w941]
                    tunnel: [w934 w939] -> w913
                    frame False {
                      n511 = Array Subset(array=w938, index (row)=0 ("index"), index (col)=0 ("index"), length (col)=w935) -> (w934:i16[][])  [unwired: 1 in]
                    }
                    frame True {
                      n512 = Array Subset(array=w942, index (row)=0 ("index"), index (col)=w941) -> (w939:i16[][])  [unwired: 2 in]
                    }
                  }
                  n513 = Array Size(array=w913) -> (size(s)=w915:i32[])
                  n514 = Transpose 2D Array(2D array=w913) -> (transposed array=w930:i16[][])
                  n515 = Multiply Array Elements(1:w915) -> (0:w931:i32)
                  n516 = Reshape Array(w930, w931) -> (w914:i16[])
                  n517 = call "write_data.vi"("Data"=w914, "Root Path"="Output Path", "N Files In"=w932, "Bird Name"="Bird Name", "RefNum In"=w929, "File Open In"="File Open?") -> ("N Files Out"=→"N Files":i16, "File Open Out"=w927:bool, "Output File Path"=→"Current File":path, "RefNum Out"=→"Outfile RefNum":refnum<file>)
                  n518 = local write "File Open?"(w927) -> ()
                  n519 = Array Size(array=w914) -> (size(s)=w921:i32)
                  n520 = Add(x=w920, y=w921) -> (x+y=w922:i32)
                }
                "First Dat" <- FALSE ("First Dat")
              }
            }
            n521 = local read "FreqVals"() -> (w851:dbl[])
            n522 = call "TAF_amp.vi"("Counters In"=w872, "Counter Rng"="Counter Rng", "AmpClust"="AmpClust", "Freq Values"=w851, "Templates"=w869, "Amp Array"=w844, "In Data"=w886, "FreqClust"="FreqClust", "Thresholds"="FFT Thresholds") -> ("LeftOverAmp"=w842:i16[], "Left Over"=w843:i16[], "Array"=w839:dbl[], "Counters Out"=w873:u32[], "Targ Syll Freq"=w840:dbl, "NoteDetect"=w848:bool, "Trigger"=w858:bool)
            "Trigger" <- w858
            "Targ Syll Freq (Hz)" <- w840
            n523 = And(x=w858, y=w883) -> (x .and. y?=w854:bool)
            n524 = local read "T Bef"() -> (w862:dbl)
            n525 = local read "Temp Out"() -> (w871:dbl[])
            n526 = Build Array (concatenate)(w871, w839) -> (w876:dbl[])
            n527 = Not(x=w854) -> (.not. x?=w857:bool)
            n528 = local write "Counters"(w873) -> ()
            n529 = And(x=w857, y=w848) -> (x .and. y?=w853:bool)
            n530 = Or(x=w835, y="Manual Trigger") -> (x .or. y?=w837:bool)
            n531 = local write "Temp Out"(w876) -> ()
            n532 = Or(x=w854, y=w837) -> (x .or. y?=w841:bool)
            n533 = Select(t=0.0, s=w853, f=w847) -> (s? t:f=w856:dbl)
            n534 = Select(t=w862, s=w864, f=w863) -> (s? t:f=w861:dbl)
            n535 = local read "Total Data T"() -> (w887:dbl)
            n536 = Add(x=w861, y=w887) -> (x+y=w860:dbl)
            n537 = case shown="True" w841 {
              tunnel: w863 -> [w972 _]
              tunnel: w860 -> [_ w994]
              tunnel: "Trig Refrac(s)" -> [w957 _]
              tunnel: w856 -> [w967 _]
              tunnel: w848 -> [w954 _]
              tunnel: w847 -> [w958 _]
              tunnel: w840 -> [_ w993]
              tunnel: w834 -> [_ w992]
              frame False {
                n538 = Add(x=w967, y=w972) -> (x+y=w970:dbl)
                n539 = local read "RecSigs"() -> (w948:bool[])
                n540 = Less Or Equal?(x=w957, y=w958) -> (x <= y?=w951:bool)
                n541 = local write "T snc trig"(w970) -> ()
                n542 = local read "N Detect"() -> (w963:i32)
                n543 = local read "DOtask"() -> (w950:refnum<k21>)
                n544 = Less Or Equal?(x=w957, y=w970) -> (x <= y?=w964:bool)
                n545 = And(x=w954, y=w951) -> (x .and. y?=w956:bool)
                n546 = Build Array (concatenate)(FALSE, w948) -> (w949:bool[])
                n547 = local read "Catch Trial?"() -> (w955:bool)
                n548 = local read "AO Started?"() -> (w968:bool)
                n549 = And(x=w954, y=w955) -> (x .and. y?=w953:bool)
                n550 = Select(t=1, s=w956, f=0) -> (s? t:f=w962:i32)
                n551 = Add(x=w962, y=w963) -> (x+y=w961:i32)
                n552 = local write "N Detect"(w961) -> ()
                n553 = And(x=w951, y=w953) -> (x .and. y?=w952:bool)
                n554 = call-poly <vilib>:"DAQmx Write.vi"("task/channels in"=w950, "data"=w949) -> ()  [unwired: 11 in, 3 out]
                n555 = local read "AO Error"() -> (w965:errorcluster)
                n556 = local read "AO task"() -> (w966:refnum<k21>)
                n557 = Not(x=w968) -> (.not. x?=w971:bool)
                n558 = case shown="True" w952 {
                  selector: w952 -> [_ w973]
                  frame False {
                  }
                  frame True {
                    n559 = flat-sequence {
                      tunnel: w973 -> [w974]
                      frame #0 {
                        n560 = local read "N Catch Esc"() -> (w976:i16)
                        n561 = Boolean To (0,1)(Boolean=w974) -> (0, 1=w975:i16)
                        n562 = Add(x=w975, y=w976) -> (x+y=→"N Catch Esc":i16)
                      }
                      frame #1 {
                        n563 = Random Number (0-1)() -> (number: 0 to 1=w980:dbl)
                        n564 = local read "Catch Trial\nFraction"() -> (w979:dbl)
                        n565 = Less Or Equal?(x=w980, y=w979) -> (x <= y?=w978:bool)
                        n566 = local write "Catch Trial?"(w978) -> ()
                      }
                    }
                  }
                }
                n567 = And(x=w971, y=w964) -> (x .and. y?=w969:bool)
                n568 = case shown="True" w969 {
                  tunnel: w966 -> [_ w983]
                  tunnel: w965 -> [_ w981]
                  frame False {
                  }
                  frame True {
                    n569 = call <vilib>:"DAQmx Is Task Done.vi"("task/channels in"=w983, "error in"=w981) -> ("task out"=w985:refnum<k21>, "task done?"=w982:bool, "error out"=w984:errorcluster)  [unwired: 11 in]
                    n570 = case shown="True" w982 {
                      tunnel: w985 -> [_ w990]
                      tunnel: w984 -> [_ w988]
                      frame False {
                      }
                      frame True {
                        n571 = call <vilib>:"DAQmx Stop Task.vi"("task/channels in"=w990, "error in"=w988) -> ("task out"=w989:refnum<k21>, "error out"=w986:errorcluster)  [unwired: 12 in]
                        "Reset Trig Error 2" <- w986
                        n572 = call <vilib>:"DAQmx Start Task.vi"("task/channels in"=w989, "error in"=w986) -> ("error out"=w987:errorcluster)  [unwired: 12 in, 1 out]
                        n573 = local write "AO Started?"(TRUE) -> ()
                        n574 = local write "AO Error"(w987) -> ()
                      }
                    }
                  }
                }
              }
              frame True {
                # "This occurrence will reset the UDP trigger variable and allow the UDPtrigger.vi to reset and look for new incoming packets."
                n575 = stacked-sequence {
                  tunnel: w994 -> [_ w1025 _ _]
                  tunnel: w993 -> [_ w1009 _ _]
                  frame #0 {
                    n576 = local read "AO Started?"() -> (w995:bool)
                    n577 = case shown="False" w995 {
                      frame False {
                        n578 = local read "AO Error"() -> (w1000:errorcluster)
                        n579 = local read "AO task"() -> (w999:refnum<k21>)
                        n580 = call <vilib>:"DAQmx Is Task Done.vi"("task/channels in"=w999, "error in"=w1000) -> ("task out"=w998:refnum<k21>, "task done?"=w996:bool, "error out"=w997:errorcluster)  [unwired: 11 in]
                        n581 = case shown="True" w996 {
                          tunnel: w998 -> [_ w1003]
                          tunnel: w997 -> [_ w1002]
                          frame False {
                          }
                          frame True {
                            n582 = call <vilib>:"DAQmx Stop Task.vi"("task/channels in"=w1003, "error in"=w1002) -> ("task out"=w1006:refnum<k21>, "error out"=w1004:errorcluster)  [unwired: 12 in]
                            "Reset Trig Error1" <- w1004
                            n583 = call <vilib>:"DAQmx Start Task.vi"("task/channels in"=w1006, "error in"=w1004) -> ("error out"=→"AO Error":errorcluster)  [unwired: 12 in, 1 out]
                            "AO Started?" <- TRUE ("Tirg Last It")
                          }
                        }
                      }
                      frame True {
                      }
                    }
                  }
                  frame #1 {
                    n584 = local read "Catch Song?"() -> (w1019:bool)
                    n585 = local read "Catch Trial?"() -> (w1018:bool)
                    n586 = local read "Syll Freqs"() -> (w1007:dbl[])
                    n587 = Build Array (concatenate)(w1007, w1009) -> (→"Syll Freqs":dbl[])
                    n588 = local read "Catch?"() -> (w1017:i32[])
                    n589 = Or(x=w1019, y=w1018) -> (x .or. y?=w1016:bool)
                    n590 = Select(t=1, s=w1016, f=0) -> (s? t:f=w1013:i32)
                    n591 = case shown="False" w1016 {
                      frame False {
                        n592 = local read "RecSigs"() -> (w1027:bool[])
                        n593 = local read "DOtask"() -> (w1030:refnum<k21>)
                        n594 = Build Array (concatenate)(TRUE, w1027) -> (w1026:bool[])
                        n595 = call-poly <vilib>:"DAQmx Write.vi"("task/channels in"=w1030, "data"=w1026) -> ()  [unwired: 11 in, 3 out]
                        n596 = call <vilib>:"High Resolution Polling Wait.vi"("seconds to wait"=0.0002) -> ()  [unwired: 10 in, 1 out]
                      }
                      frame True {
                        n597 = local read "RecSigs"() -> (w1032:bool[])
                        n598 = local read "DOtask"() -> (w1034:refnum<k21>)
                        n599 = Build Array (concatenate)(FALSE, w1032) -> (w1031:bool[])
                        n600 = call-poly <vilib>:"DAQmx Write.vi"("task/channels in"=w1034, "data"=w1031) -> ()  [unwired: 11 in, 3 out]
                      }
                    }
                    n601 = Build Array (concatenate)(w1017, w1013) -> (→"Catch?":i32[])
                    n602 = local read "Trig Times"() -> (w1022:dbl[])
                    n603 = Build Array (concatenate)(w1022, w1025) -> (→"Trig Times":dbl[])
                    n604 = local read "N Detect"() -> (w1011:i32)
                    n605 = local read "N Trig"() -> (w1021:u32)
                    n606 = Increment(x=w1021) -> (x+1=→"N Trig":u32)
                    n607 = Increment(x=w1011) -> (x+1=→"N Detect":i32)
                    "T snc trig" <- 0.0 ("T snc trig")
                  }
                  frame #2 {
                    n608 = local read "Catch Song?"() -> (w1036:bool)
                    n609 = local read "Catch Trial?"() -> (w1037:bool)
                    n610 = local write "Manual Trigger"(FALSE ("Manual Trigger")) -> ()
                    n611 = Or(x=w1036, y=w1037) -> (x .or. y?=w1035:bool)
                    n612 = case shown="True" w1035 {
                      frame False {
                        n613 = local read "RecSigs"() -> (w1039:bool[])
                        n614 = local read "DOtask"() -> (w1043:refnum<k21>)
                        n615 = Build Array (concatenate)(FALSE, w1039) -> (w1040:bool[])
                        n616 = local write "AO Started?"(FALSE ("AO Started?")) -> ()
                        n617 = call-poly <vilib>:"DAQmx Write.vi"("task/channels in"=w1043, "auto start"=FALSE ("data"), "data"=w1040) -> ()  [unwired: 10 in, 3 out]
                      }
                      frame True {
                        n618 = local read "RecSigs"() -> (w1046:bool[])
                        n619 = local read "DOtask"() -> (w1048:refnum<k21>)
                        n620 = Build Array (concatenate)(FALSE, w1046) -> (w1045:bool[])
                        n621 = call-poly <vilib>:"DAQmx Write.vi"("task/channels in"=w1048, "auto start"=FALSE, "data"=w1045) -> ()  [unwired: 10 in, 3 out]
                      }
                    }
                  }
                  frame #3 {
                    n622 = Random Number (0-1)() -> (number: 0 to 1=w1052:dbl)
                    n623 = Less Or Equal?(x=w1052, y="Catch Trial\nFraction") -> (x <= y?=→"Catch Trial?":bool)
                  }
                }
                n624 = Set Occurrence(w992) -> ()
              }
            }
            n625 = case shown="True" w841 {
              frame False {
              }
              frame True {
                n626 = Tick Count (ms)() -> (millisecond timer value=→"Trig Time":u32)
              }
            }
            n627 = local read "N AI Chan"() -> (w867:i32)
            n628 = To Double Precision Float(number=w868) -> (double precision float=w866:dbl)
            n629 = Divide(x=w866, y=w867) -> (x/y=w882:dbl)
            n630 = Round To Nearest(number=w882) -> (nearest integer value=w881:dbl)
            n631 = To Long Integer(number=w881) -> (32bit integer=w878:i32)
            n632 = Add(x=w878, y=w880) -> (x+y=w879:i32)
          }
        }
        "Total Data T" <- w611
        n633 = local read "DOtask"() -> (w616:refnum<k21>)
        "Silence T" <- w604
      }
      n634 = call <vilib>:"DAQmx Clear Task.vi"("task in"=w478, "error in"=w510) -> ("error out"=w509:errorcluster)  [unwired: 13 in]
      n635 = local write "AI Error"(w509) -> ()
      n636 = call <vilib>:"DAQmx Clear Task.vi"("task in"=w486, "error in"=w485) -> ("error out"=w484:errorcluster)  [unwired: 13 in]
      n637 = local write "AO Error"(w484) -> ()
      n638 = call <vilib>:"DAQmx Clear Task.vi"("task in"=w479) -> ()  [unwired: 14 in, 1 out]
    }
  }
